vi "Main.vi"(10 "Ip-Address":string="192.168.81.153", 11 "Module Admin":refnum<class "Delacor_lib_QMH_Cloneable Module Admin.lvclass">) -> ()   [LabVIEW 2021, in "RT Acquisition Engine.lvlib"]
doc: "This template is based off of the Queued Message Handler design pattern and the Queued Message Handler project template that ships with LabVIEW.\n\nThe main difference is that the queue is private to this module and communication between modules is performed via Broadcast and Request events.\n\nRequest events are wrapped in public API methods and are handled in the Event Handling Loop (EHL) of this VI. Any module can register for Broadcast events sent by this module. The EHL generates messages based on user interface actions.\n\nThe Message Handling Loop (MHL) processes messages generated by the EHL, or by other messages. The messages are string values, so new messages can be added easily to the Message Cases case structure in the MHL. Each message cluster can also provide an optional value for Message Data, which is a variant that can be converted to whatever message-specific data is required.\n_____\nBased on DQMH Project Template 7.0.1.1316."
uses:
  RT Acquisition Engine.lvlib
  <vilib>/Delacor/Delacor QMH/Libraries/Cloneable Module Admin_class/Delacor_lib_QMH_Cloneable Module Admin.lvclass
  C:/Program Files (x86)/National Instruments/LabVIEW 2024/vi.lib/Delacor/Delacor QMH/Libraries/Module Admin_class/Delacor_lib_QMH_Module Admin.lvclass
  Analog Output/Controls/AO JSON Data Cluster.ctl
  Analog Output/Controls/AO Interface Data Cluster.ctl
  Analog Output/Controls/AO Channel Configuration Cluster.ctl
  Analog Output/Controls/AO Timing Cluster.ctl
  Digital Output/Controls/DIO Configuration cluster.ctl
  Digital Output/Controls/DIO Interface Data.ctl
  Digital Output/SubVIs/Digital Dynamic Cluster.ctl
  Host/Async JSON Cluster.ctl
  Host/Async Interface Data Cluster.ctl
  Async Serial/Controls/Async Serial Configuration Cluster.ctl
  Async Serial/Controls/Async Frame Info Cluster.ctl
  Async Serial/Controls/Async Message Info Cluster.ctl
  Host-Control's/TCP Tx-Rx cluster.ctl
  Host-Control's/AI-Data from RT.ctl
  Main Engine/Controls/Main Engine Serial Info JSON Data.ctl
  Main Engine/Controls/Main Engine DAQ Harware Info JSON Data.ctl
  Main Engine/Controls/Main Engine Ehernet IP Address JSON Data.ctl
  Module Data--cluster.ctl
  Hardware Info (Reply Payload)--cluster.ctl
  Host-Control's/RT Data's.ctl
  Host-Control's/DIO Data's from RT.ctl
  <vilib>/Wovalab/Utilities/Helper Loop Periodic Timing/Helper Loop Periodic Timing.lvclass/Helper Loop Periodic Timing.ctl
  <vilib>/Delacor/Delacor QMH/Libraries/Message Queue_class/Delacor_lib_QMH_Message Queue.lvclass/Delacor_lib_QMH_Message Queue.ctl
  <vilib>/Delacor/Delacor QMH/Libraries/Cloneable Module Admin_class/Delacor_lib_QMH_Cloneable Module Admin.lvclass/Delacor_lib_QMH_Cloneable Module Admin.ctl
  Stop Argument--cluster.ctl
  <vilib>/Delacor/Delacor QMH/Libraries/Module Admin_class/Delacor_lib_QMH_Module Admin.lvclass/Delacor_lib_QMH_Module Admin.ctl
  Write Data To the RT Argument--cluster.ctl
  <vilib>/Utility/miscctls.llb/LVPointTypeDef.ctl
  <vilib>/Delacor/Delacor QMH/Libraries/Message Queue_class/Delacor_lib_QMH_Enqueue Message (Single).vi
  <vilib>/Delacor/Delacor QMH/Libraries/Cloneable Module Admin_class/Delacor_lib_QMH_Get Module ID.vi
  <vilib>/Delacor/Delacor QMH/Libraries/Module Admin_class/Delacor_lib_QMH_Get External Launch.vi
  <vilib>/Wovalab/Utilities/Helper Loop Periodic Timing/U32 Max Value--constant.vi
  <vilib>/Wovalab/Utilities/Helper Loop Periodic Timing/Update Last Execution Time.vi
  <vilib>/Wovalab/Utilities/Helper Loop Periodic Timing/Helper Loop Periodic Timing.lvclass
  <vilib>/Delacor/Delacor QMH/Libraries/Message Queue_class/Delacor_lib_QMH_Message Queue.lvclass
  TCP-IP Engine/TCP-IP Engine.lvlib
  <vilib>/addons/_JKI.lib/Serialization/JSON/JKI JSON Serialization.lvlib
panel:
  in  "AI-Info":T1
  out "TCP-IP Data Out 2":string
  out "Connection Status?":bool
  out "TCP-IP Module ID":i32
  out "data":T2={"Interface"="CPU", "Command"="CPU Info", "SubCmd"="Monitor", "Data"=variant}
  in  "DO":T3={"Interface"="DIO", "Interface Data"={"Command"="Configure", "SubCmd"="DO", "Frequency"=500, "Data"=[{"Channel"="Mod1/port0/line0", "Data"=[0], "Identification Name"=""}, {"Channel"="Mod1/port0/line1", "Data"=[0], "Identification Name"=""}, {"Channel"="Mod1/port0/line2", "Data"=[0], "Identification Name"=""}, {"Channel"="Mod1/port0/line3", "Data"=[0], "Identification Name"=""}, {"Channel"="Mod1/port0/line4", "Data"=[0], "Identification Name"=""}, {"Channel"="Mod1/port0/line5", "Data"=[0], "Identification Name"=""}, {"Channel"="Mod1/port0/line6", "Data"=[0], "Identification Name"=""}, {"Channel"="Mod1/port0/line7", "Data"=[0], "Identification Name"=""}, {"Channel"="Mod1/port0/line8", "Data"=[0], "Identification Name"=""}, {"Channel"="Mod1/port0/line9", "Data"=[0], "Identification Name"=""}, {"Channel"="Mod1/port0/line10", "Data"=[0], "Identification Name"=""}, {"Channel"="Mod1/port0/line11", "Data"=[0], "Identification Name"=""}, {"Channel"="Mod1/port0/line12", "Data"=[0], "Identification Name"=""}, {"Channel"="Mod1/port0/line13", "Data"=[0], "Identification Name"=""}, {"Channel"="Mod1/port0/line14", "Data"=[0], "Identification Name"=""}, {"Channel"="Mod1/port0/line15", "Data"=[0], "Identification Name"=""}, {"Channel"="Mod1/port0/line16", "Data"=[0], "Identification Name"=""}, {"Channel"="Mod1/port0/line17", "Data"=[0], "Identification Name"=""}, {"Channel"="Mod1/port0/line18", "Data"=[0], "Identification Name"=""}, {"Channel"="Mod1/port0/line19", "Data"=[0], "Identification Name"=""}, {"Channel"="Mod1/port0/line20", "Data"=[0], "Identification Name"=""}, {"Channel"="Mod1/port0/line21", "Data"=[0], "Identification Name"=""}, {"Channel"="Mod1/port0/line22", "Data"=[0], "Identification Name"=""}, {"Channel"="Mod1/port0/line23", "Data"=[0], "Identification Name"=""}, {"Channel"="Mod1/port0/line24", "Data"=[0], "Identification Name"=""}, {"Channel"="Mod1/port0/line25", "Data"=[0], "Identification Name"=""}, {"Channel"="Mod1/port0/line26", "Data"=[0], "Identification Name"=""}, {"Channel"="Mod1/port0/line27", "Data"=[0], "Identification Name"=""}, {"Channel"="Mod1/port0/line28", "Data"=[0], "Identification Name"=""}, {"Channel"="Mod1/port0/line29", "Data"=[0], "Identification Name"=""}, {"Channel"="Mod1/port0/line30", "Data"=[0], "Identification Name"=""}, {"Channel"="Mod1/port0/line31", "Data"=[0], "Identification Name"=""}]}}
  in  "Channel Data":cluster{"AI":T6, "DI":T3, "DO":T3, "Async":T10}={"AI"={"Interface"="AIO", "Interface Data"={"Command"="Configure", "SubCmd"="AI", "Data"=[{"Channel"="Mod2/ai0", "Min Value"=-5.0, "Max Value"=5.0, "Type"="Voltage", "Terminal Configure"=10083, "Dynamic"=0, "Dyn Type"="", "Data"=[], "File Name"="", "Column"=0, "Frequency"=0.0}, {"Channel"="Mod2/ai1", "Min Value"=-5.0, "Max Value"=5.0, "Type"="Voltage", "Terminal Configure"=10083, "Dynamic"=0, "Dyn Type"="", "Data"=[], "File Name"="", "Column"=0, "Frequency"=0.0}, {"Channel"="Mod2/ai2", "Min Value"=-5.0, "Max Value"=5.0, "Type"="Voltage", "Terminal Configure"=10083, "Dynamic"=0, "Dyn Type"="", "Data"=[], "File Name"="", "Column"=0, "Frequency"=0.0}, {"Channel"="Mod2/ai3", "Min Value"=-5.0, "Max Value"=5.0, "Type"="Voltage", "Terminal Configure"=10083, "Dynamic"=0, "Dyn Type"="", "Data"=[], "File Name"="", "Column"=0, "Frequency"=0.0}, {"Channel"="Mod2/ai4", "Min Value"=-5.0, "Max Value"=5.0, "Type"="Voltage", "Terminal Configure"=10083, "Dynamic"=0, "Dyn Type"="", "Data"=[], "File Name"="", "Column"=0, "Frequency"=0.0}, {"Channel"="Mod2/ai5", "Min Value"=-5.0, "Max Value"=5.0, "Type"="Voltage", "Terminal Configure"=10083, "Dynamic"=0, "Dyn Type"="", "Data"=[], "File Name"="", "Column"=0, "Frequency"=0.0}, {"Channel"="Mod2/ai6", "Min Value"=-5.0, "Max Value"=5.0, "Type"="Voltage", "Terminal Configure"=10083, "Dynamic"=0, "Dyn Type"="", "Data"=[], "File Name"="", "Column"=0, "Frequency"=0.0}, {"Channel"="Mod2/ai7", "Min Value"=-5.0, "Max Value"=5.0, "Type"="Voltage", "Terminal Configure"=10083, "Dynamic"=0, "Dyn Type"="", "Data"=[], "File Name"="", "Column"=0, "Frequency"=0.0}, {"Channel"="Mod2/ai8", "Min Value"=-5.0, "Max Value"=5.0, "Type"="Voltage", "Terminal Configure"=10083, "Dynamic"=0, "Dyn Type"="", "Data"=[], "File Name"="", "Column"=0, "Frequency"=0.0}, {"Channel"="Mod2/ai9", "Min Value"=-5.0, "Max Value"=5.0, "Type"="Voltage", "Terminal Configure"=10083, "Dynamic"=0, "Dyn Type"="", "Data"=[], "File Name"="", "Column"=0, "Frequency"=0.0}, {"Channel"="Mod2/ai10", "Min Value"=-5.0, "Max Value"=5.0, "Type"="Voltage", "Terminal Configure"=10083, "Dynamic"=0, "Dyn Type"="", "Data"=[], "File Name"="", "Column"=0, "Frequency"=0.0}, {"Channel"="Mod2/ai11", "Min Value"=-5.0, "Max Value"=5.0, "Type"="Voltage", "Terminal Configure"=10083, "Dynamic"=0, "Dyn Type"="", "Data"=[], "File Name"="", "Column"=0, "Frequency"=0.0}, {"Channel"="Mod2/ai12", "Min Value"=-5.0, "Max Value"=5.0, "Type"="Voltage", "Terminal Configure"=10083, "Dynamic"=0, "Dyn Type"="", "Data"=[], "File Name"="", "Column"=0, "Frequency"=0.0}, {"Channel"="Mod2/ai13", "Min Value"=-5.0, "Max Value"=5.0, "Type"="Voltage", "Terminal Configure"=10083, "Dynamic"=0, "Dyn Type"="", "Data"=[], "File Name"="", "Column"=0, "Frequency"=0.0}, {"Channel"="Mod2/ai14", "Min Value"=-5.0, "Max Value"=5.0, "Type"="Voltage", "Terminal Configure"=10083, "Dynamic"=0, "Dyn Type"="", "Data"=[], "File Name"="", "Column"=0, "Frequency"=0.0}, {"Channel"="Mod2/ai15", "Min Value"=-5.0, "Max Value"=5.0, "Type"="Voltage", "Terminal Configure"=10083, "Dynamic"=0, "Dyn Type"="", "Data"=[], "File Name"="", "Column"=0, "Frequency"=0.0}, {"Channel"="Mod2/ai16", "Min Value"=-5.0, "Max Value"=5.0, "Type"="Voltage", "Terminal Configure"=10083, "Dynamic"=0, "Dyn Type"="", "Data"=[], "File Name"="", "Column"=0, "Frequency"=0.0}, {"Channel"="Mod2/ai17", "Min Value"=-5.0, "Max Value"=5.0, "Type"="Voltage", "Terminal Configure"=10083, "Dynamic"=0, "Dyn Type"="", "Data"=[], "File Name"="", "Column"=0, "Frequency"=0.0}, {"Channel"="Mod2/ai18", "Min Value"=-5.0, "Max Value"=5.0, "Type"="Voltage", "Terminal Configure"=10083, "Dynamic"=0, "Dyn Type"="", "Data"=[], "File Name"="", "Column"=0, "Frequency"=0.0}, {"Channel"="Mod2/ai19", "Min Value"=-5.0, "Max Value"=5.0, "Type"="Voltage", "Terminal Configure"=10083, "Dynamic"=0, "Dyn Type"="", "Data"=[], "File Name"="", "Column"=0, "Frequency"=0.0}, {"Channel"="Mod2/ai20", "Min Value"=-5.0, "Max Value"=5.0, "Type"="Voltage", "Terminal Configure"=10083, "Dynamic"=0, "Dyn Type"="", "Data"=[], "File Name"="", "Column"=0, "Frequency"=0.0}, {"Channel"="Mod2/ai21", "Min Value"=-5.0, "Max Value"=5.0, "Type"="Voltage", "Terminal Configure"=10083, "Dynamic"=0, "Dyn Type"="", "Data"=[], "File Name"="", "Column"=0, "Frequency"=0.0}, {"Channel"="Mod2/ai22", "Min Value"=-5.0, "Max Value"=5.0, "Type"="Voltage", "Terminal Configure"=10083, "Dynamic"=0, "Dyn Type"="", "Data"=[], "File Name"="", "Column"=0, "Frequency"=0.0}, {"Channel"="Mod2/ai23", "Min Value"=-5.0, "Max Value"=5.0, "Type"="Voltage", "Terminal Configure"=10083, "Dynamic"=0, "Dyn Type"="", "Data"=[], "File Name"="", "Column"=0, "Frequency"=0.0}, {"Channel"="Mod2/ai24", "Min Value"=-5.0, "Max Value"=5.0, "Type"="Voltage", "Terminal Configure"=10083, "Dynamic"=0, "Dyn Type"="", "Data"=[], "File Name"="", "Column"=0, "Frequency"=0.0}, {"Channel"="Mod2/ai25", "Min Value"=-5.0, "Max Value"=5.0, "Type"="Voltage", "Terminal Configure"=10083, "Dynamic"=0, "Dyn Type"="", "Data"=[], "File Name"="", "Column"=0, "Frequency"=0.0}, {"Channel"="Mod2/ai26", "Min Value"=-5.0, "Max Value"=5.0, "Type"="Voltage", "Terminal Configure"=10083, "Dynamic"=0, "Dyn Type"="", "Data"=[], "File Name"="", "Column"=0, "Frequency"=0.0}, {"Channel"="Mod2/ai27", "Min Value"=-5.0, "Max Value"=5.0, "Type"="Voltage", "Terminal Configure"=10083, "Dynamic"=0, "Dyn Type"="", "Data"=[], "File Name"="", "Column"=0, "Frequency"=0.0}, {"Channel"="Mod2/ai28", "Min Value"=-5.0, "Max Value"=5.0, "Type"="Voltage", "Terminal Configure"=10083, "Dynamic"=0, "Dyn Type"="", "Data"=[], "File Name"="", "Column"=0, "Frequency"=0.0}, {"Channel"="Mod2/ai29", "Min Value"=-5.0, "Max Value"=5.0, "Type"="Voltage", "Terminal Configure"=10083, "Dynamic"=0, "Dyn Type"="", "Data"=[], "File Name"="", "Column"=0, "Frequency"=0.0}, {"Channel"="Mod2/ai30", "Min Value"=-5.0, "Max Value"=5.0, "Type"="Voltage", "Terminal Configure"=10083, "Dynamic"=0, "Dyn Type"="", "Data"=[], "File Name"="", "Column"=0, "Frequency"=0.0}, {"Channel"="Mod2/ai31", "Min Value"=-5.0, "Max Value"=5.0, "Type"="Voltage", "Terminal Configure"=65535, "Dynamic"=0, "Dyn Type"="", "Data"=[], "File Name"="", "Column"=0, "Frequency"=0.0}], "Timing"={"samples per channel"=4, "sample mode"=10123, "Sampling Rate"=2.0}}}, "DI"={"Interface"="DIO", "Interface Data"={"Command"="Configure", "SubCmd"="DI", "Frequency"=500, "Data"=[{"Channel"="Mod3/port0/line0", "Data"=[0], "Identification Name"=""}, {"Channel"="Mod3/port0/line1", "Data"=[0], "Identification Name"=""}, {"Channel"="Mod3/port0/line2", "Data"=[0], "Identification Name"=""}, {"Channel"="Mod3/port0/line3", "Data"=[0], "Identification Name"=""}, {"Channel"="Mod3/port0/line4", "Data"=[0], "Identification Name"=""}, {"Channel"="Mod3/port0/line5", "Data"=[0], "Identification Name"=""}, {"Channel"="Mod3/port0/line6", "Data"=[0], "Identification Name"=""}, {"Channel"="Mod3/port0/line7", "Data"=[0], "Identification Name"=""}, {"Channel"="Mod3/port0/line8", "Data"=[0], "Identification Name"=""}, {"Channel"="Mod3/port0/line9", "Data"=[0], "Identification Name"=""}, {"Channel"="Mod3/port0/line10", "Data"=[0], "Identification Name"=""}, {"Channel"="Mod3/port0/line11", "Data"=[0], "Identification Name"=""}, {"Channel"="Mod3/port0/line12", "Data"=[0], "Identification Name"=""}, {"Channel"="Mod3/port0/line13", "Data"=[0], "Identification Name"=""}, {"Channel"="Mod3/port0/line14", "Data"=[0], "Identification Name"=""}, {"Channel"="Mod3/port0/line15", "Data"=[0], "Identification Name"=""}, {"Channel"="Mod3/port0/line16", "Data"=[0], "Identification Name"=""}, {"Channel"="Mod3/port0/line17", "Data"=[0], "Identification Name"=""}, {"Channel"="Mod3/port0/line18", "Data"=[0], "Identification Name"=""}, {"Channel"="Mod3/port0/line19", "Data"=[0], "Identification Name"=""}, {"Channel"="Mod3/port0/line20", "Data"=[0], "Identification Name"=""}, {"Channel"="Mod3/port0/line21", "Data"=[0], "Identification Name"=""}, {"Channel"="Mod3/port0/line22", "Data"=[0], "Identification Name"=""}, {"Channel"="Mod3/port0/line23", "Data"=[0], "Identification Name"=""}, {"Channel"="Mod3/port0/line24", "Data"=[0], "Identification Name"=""}, {"Channel"="Mod3/port0/line25", "Data"=[0], "Identification Name"=""}, {"Channel"="Mod3/port0/line26", "Data"=[0], "Identification Name"=""}, {"Channel"="Mod3/port0/line27", "Data"=[0], "Identification Name"=""}, {"Channel"="Mod3/port0/line28", "Data"=[0], "Identification Name"=""}, {"Channel"="Mod3/port0/line29", "Data"=[0], "Identification Name"=""}, {"Channel"="Mod3/port0/line30", "Data"=[0], "Identification Name"=""}, {"Channel"="Mod3/port0/line31", "Data"=[0], "Identification Name"=""}, {"Channel"="Mod4/port0/line0", "Data"=[0], "Identification Name"=""}, {"Channel"="Mod4/port0/line1", "Data"=[0], "Identification Name"=""}, {"Channel"="Mod4/port0/line2", "Data"=[0], "Identification Name"=""}, {"Channel"="Mod4/port0/line3", "Data"=[0], "Identification Name"=""}, {"Channel"="Mod4/port0/line4", "Data"=[0], "Identification Name"=""}, {"Channel"="Mod4/port0/line5", "Data"=[0], "Identification Name"=""}, {"Channel"="Mod4/port0/line6", "Data"=[0], "Identification Name"=""}, {"Channel"="Mod4/port0/line7", "Data"=[0], "Identification Name"=""}, {"Channel"="Mod4/port0/line8", "Data"=[0], "Identification Name"=""}, {"Channel"="Mod4/port0/line9", "Data"=[0], "Identification Name"=""}, {"Channel"="Mod4/port0/line10", "Data"=[0], "Identification Name"=""}, {"Channel"="Mod4/port0/line11", "Data"=[0], "Identification Name"=""}, {"Channel"="Mod4/port0/line12", "Data"=[0], "Identification Name"=""}, {"Channel"="Mod4/port0/line13", "Data"=[0], "Identification Name"=""}, {"Channel"="Mod4/port0/line14", "Data"=[0], "Identification Name"=""}, {"Channel"="Mod4/port0/line15", "Data"=[0], "Identification Name"=""}, {"Channel"="Mod4/port0/line16", "Data"=[0], "Identification Name"=""}, {"Channel"="Mod4/port0/line17", "Data"=[0], "Identification Name"=""}, {"Channel"="Mod4/port0/line18", "Data"=[0], "Identification Name"=""}, {"Channel"="Mod4/port0/line19", "Data"=[0], "Identification Name"=""}, {"Channel"="Mod4/port0/line20", "Data"=[0], "Identification Name"=""}, {"Channel"="Mod4/port0/line21", "Data"=[0], "Identification Name"=""}, {"Channel"="Mod4/port0/line22", "Data"=[0], "Identification Name"=""}, {"Channel"="Mod4/port0/line23", "Data"=[0], "Identification Name"=""}, {"Channel"="Mod4/port0/line24", "Data"=[0], "Identification Name"=""}, {"Channel"="Mod4/port0/line25", "Data"=[0], "Identification Name"=""}, {"Channel"="Mod4/port0/line26", "Data"=[0], "Identification Name"=""}, {"Channel"="Mod4/port0/line27", "Data"=[0], "Identification Name"=""}, {"Channel"="Mod4/port0/line28", "Data"=[0], "Identification Name"=""}, {"Channel"="Mod4/port0/line29", "Data"=[0], "Identification Name"=""}, {"Channel"="Mod4/port0/line30", "Data"=[0], "Identification Name"=""}, {"Channel"="Mod4/port0/line31", "Data"=[0], "Identification Name"=""}]}}, "DO"={"Interface"="DIO", "Interface Data"={"Command"="Configure", "SubCmd"="DO", "Frequency"=500, "Data"=[{"Channel"="Mod1/port0/line0", "Data"=[0], "Identification Name"=""}, {"Channel"="Mod1/port0/line1", "Data"=[0], "Identification Name"=""}, {"Channel"="Mod1/port0/line2", "Data"=[0], "Identification Name"=""}, {"Channel"="Mod1/port0/line3", "Data"=[0], "Identification Name"=""}, {"Channel"="Mod1/port0/line4", "Data"=[0], "Identification Name"=""}, {"Channel"="Mod1/port0/line5", "Data"=[0], "Identification Name"=""}, {"Channel"="Mod1/port0/line6", "Data"=[0], "Identification Name"=""}, {"Channel"="Mod1/port0/line7", "Data"=[0], "Identification Name"=""}, {"Channel"="Mod1/port0/line8", "Data"=[0], "Identification Name"=""}, {"Channel"="Mod1/port0/line9", "Data"=[0], "Identification Name"=""}, {"Channel"="Mod1/port0/line10", "Data"=[0], "Identification Name"=""}, {"Channel"="Mod1/port0/line11", "Data"=[0], "Identification Name"=""}, {"Channel"="Mod1/port0/line12", "Data"=[0], "Identification Name"=""}, {"Channel"="Mod1/port0/line13", "Data"=[0], "Identification Name"=""}, {"Channel"="Mod1/port0/line14", "Data"=[0], "Identification Name"=""}, {"Channel"="Mod1/port0/line15", "Data"=[0], "Identification Name"=""}, {"Channel"="Mod1/port0/line16", "Data"=[0], "Identification Name"=""}, {"Channel"="Mod1/port0/line17", "Data"=[0], "Identification Name"=""}, {"Channel"="Mod1/port0/line18", "Data"=[0], "Identification Name"=""}, {"Channel"="Mod1/port0/line19", "Data"=[0], "Identification Name"=""}, {"Channel"="Mod1/port0/line20", "Data"=[0], "Identification Name"=""}, {"Channel"="Mod1/port0/line21", "Data"=[0], "Identification Name"=""}, {"Channel"="Mod1/port0/line22", "Data"=[0], "Identification Name"=""}, {"Channel"="Mod1/port0/line23", "Data"=[0], "Identification Name"=""}, {"Channel"="Mod1/port0/line24", "Data"=[0], "Identification Name"=""}, {"Channel"="Mod1/port0/line25", "Data"=[0], "Identification Name"=""}, {"Channel"="Mod1/port0/line26", "Data"=[0], "Identification Name"=""}, {"Channel"="Mod1/port0/line27", "Data"=[0], "Identification Name"=""}, {"Channel"="Mod1/port0/line28", "Data"=[0], "Identification Name"=""}, {"Channel"="Mod1/port0/line29", "Data"=[0], "Identification Name"=""}, {"Channel"="Mod1/port0/line30", "Data"=[0], "Identification Name"=""}, {"Channel"="Mod1/port0/line31", "Data"=[0], "Identification Name"=""}]}}, "Async"={"Interface"="Async", "Interface Data"={"Command"="Configure", "SubCmd"="Async", "Data"=[{"Port"="com10", "Minor Frame Freq"=200, "Minor Frame Count"=1, "Frame Info"=[{"Frame ID"=1, "Message Info"=[{"Message"=[1], "Message Name"="m1"}]}], "Sensor Type"=0, "OIM Address"=0}]}}} {"Async"."Interface Data"."Data"."Minor Frame Count" min=5 max=8 step=1; "AI"."Interface Data"."Timing"."sample mode" items=["Finite Samples"=10178, "Continuous Samples"=10123, "Hardware Timed Single Point"=12522]}
  out "error out":errorcluster
  out "Status":string
  in  "Simulate EHL Error":bool
  in  "Simulate MHL Error":bool
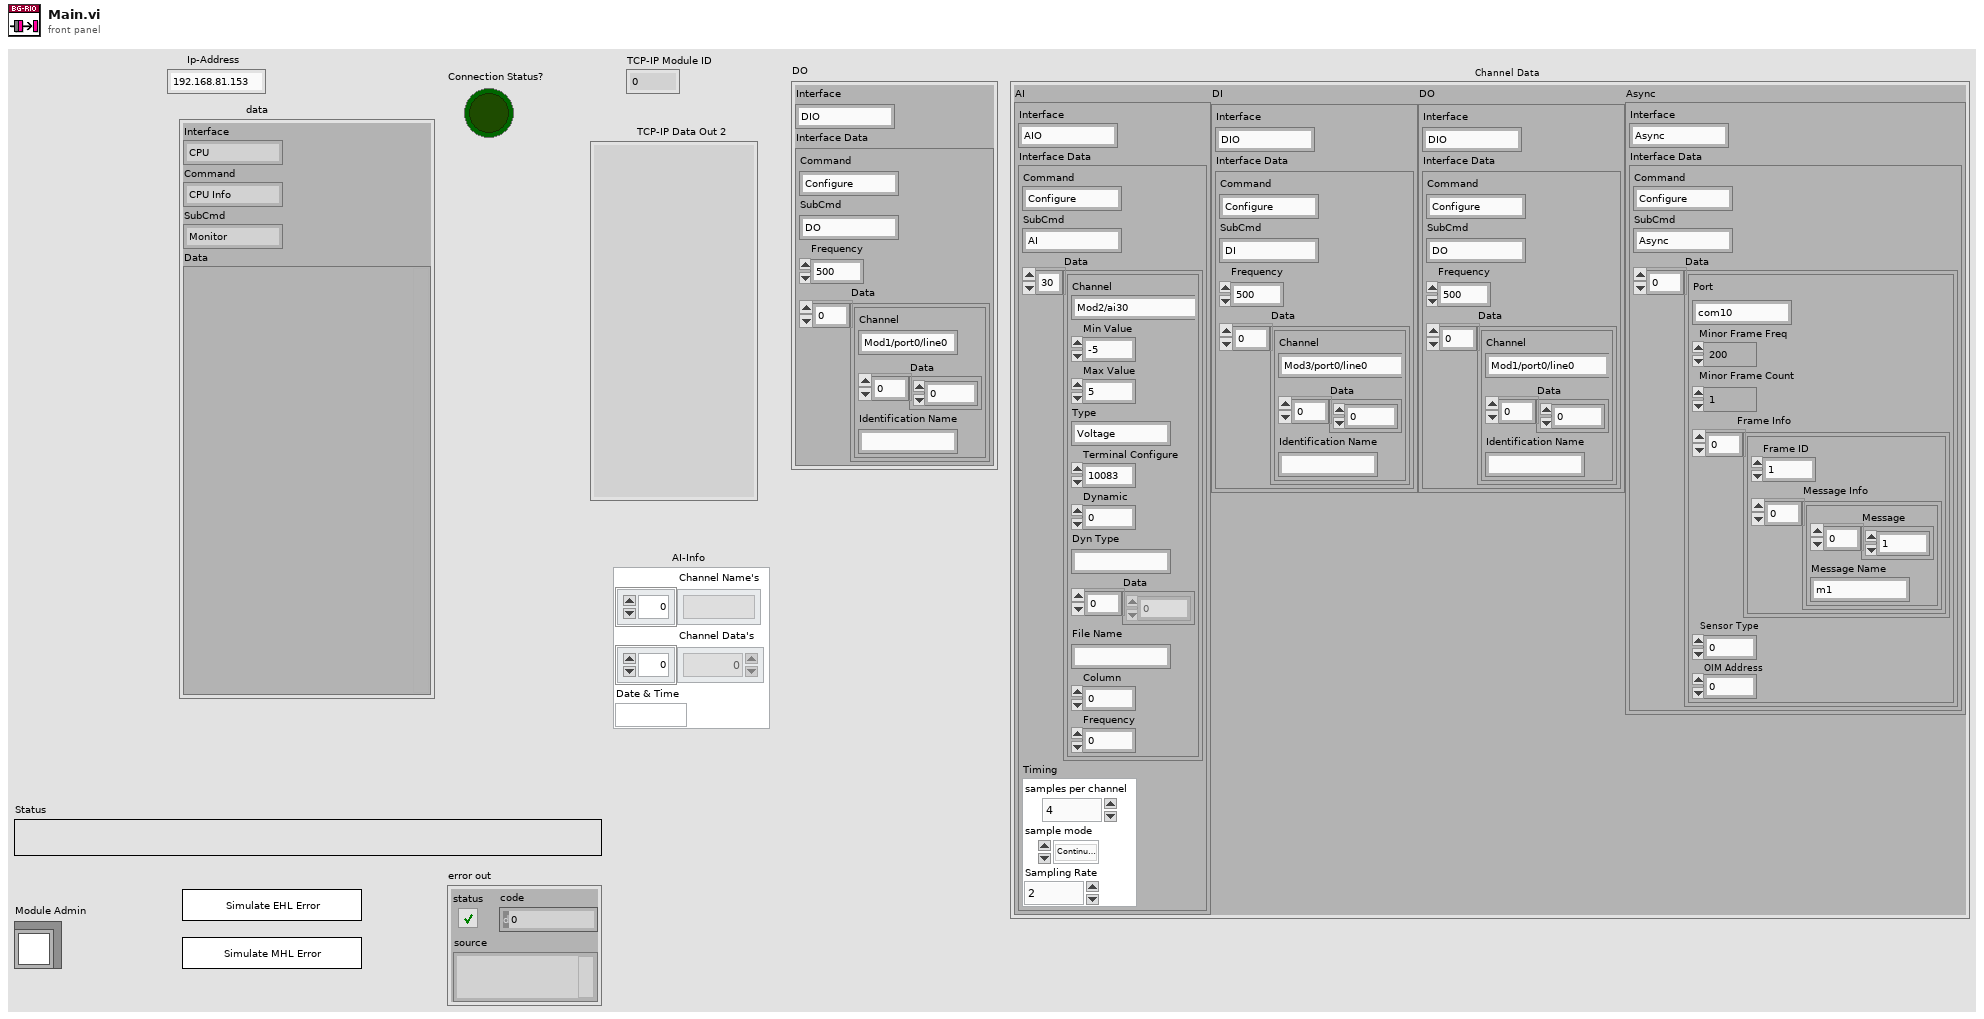
[diagram p1: front panel]
types:
  T1 = typedef "AI-Data from RT.ctl" = cluster{"Channel Name's":string[], "Channel Data's":dbl[], "Date & Time":string}
  T2 = typedef "TCP Tx-Rx cluster.ctl" = cluster{"Interface":string, "Command":string, "SubCmd":string, "Data":variant}
  T3 = typedef "DIO Configuration cluster.ctl" = cluster{"Interface":string, "Interface Data":T4}
  T4 = typedef "DIO Interface Data.ctl" = cluster{"Command":string, "SubCmd":string, "Frequency":u16, "Data":T5[]}
  T5 = typedef "Digital Dynamic Cluster.ctl" = cluster{"Channel":string, "Data":u8[], "Identification Name":string}
  T6 = typedef "AO JSON Data Cluster.ctl" = cluster{"Interface":string, "Interface Data":T7}
  T7 = typedef "AO Interface Data Cluster.ctl" = cluster{"Command":string, "SubCmd":string, "Data":T8[], "Timing":T9}
  T8 = typedef "AO Channel Configuration Cluster.ctl" = cluster{"Channel":string, "Min Value":dbl, "Max Value":dbl, "Type":string, "Terminal Configure":u16, "Dynamic":u8, "Dyn Type":string, "Data":dbl[], "File Name":string, "Column":i32, "Frequency":dbl}
  T9 = typedef "AO Timing Cluster.ctl" = cluster{"samples per channel":i32, "sample mode":i32, "Sampling Rate":dbl}
  T10 = typedef "Async JSON Cluster.ctl" = cluster{"Interface":string, "Interface Data":T11}
  T11 = typedef "Async Interface Data Cluster.ctl" = cluster{"Command":string, "SubCmd":string, "Data":T12[]}
  T12 = typedef "Async Serial Configuration Cluster.ctl" = cluster{"Port":string, "Minor Frame Freq":u16, "Minor Frame Count":u16, "Frame Info":T13[], "Sensor Type":u16, "OIM Address":u16}
  T13 = typedef "Async Frame Info Cluster.ctl" = cluster{"Frame ID":u16, "Message Info":T14[]}
  T14 = typedef "Async Message Info Cluster.ctl" = cluster{"Message":u8[], "Message Name":string}
  T15 = typedef "Main Engine Serial Info JSON Data.ctl" = cluster{"Command":string, "SubCmd":string, "Channel":string[]}
  T16 = typedef "Main Engine DAQ Harware Info JSON Data.ctl" = cluster{"Command":string, "SubCmd":string, "Input":string[], "Output":string[]}
  T17 = typedef "Main Engine Ehernet IP Address JSON Data.ctl" = cluster{"Command":string, "SubCmd":string, "IP":string[]}
  T18 = cluster{"Serial Hardware Info JSON Format":T15, "Hardware Info JSON Format":T16, "Hardware Info JSON Format":T16, "Ethernet IP Address JSON Format":T17}
  T19 = typedef "RT Acquisition Engine.lvlib/Request Events--cluster.ctl" = cluster{"Stop Module":refnum<user-event>, "Show Panel":refnum<user-event>, "Hide Panel":refnum<user-event>, "Show Diagram":refnum<user-event>, "Get Module Execution Status":refnum<user-event>, "Write Data To the RT":refnum<user-event>, "Hardware Info":refnum<user-event>}
  T20 = enum16{"Standard", "Buffered", "CRLF", "Immediate"}
  T21 = enum32{"invalid lock state", "Not Locked", "Locked (No Password)", "Password-protected"}
  T22 = typedef "RT Acquisition Engine.lvlib/Stop Argument--cluster.ctl" = cluster{"Module ID":i32, "Origin":string, "Exit via Stop Module Req?":bool, "Wait for Module to stop?":bool}
  T23 = typedef "RT Acquisition Engine.lvlib/Write Data To the RT Argument--cluster.ctl" = cluster{"Module ID":i32, "Data In":string}
  T24 = typedef "LVPointTypeDef.ctl" = cluster{"Horizontal":i16, "Vertical":i16}
  T25 = enum32{"Invalid", "Standard", "Closed", "Hidden", "Minimized", "Maximized"}
  T26 = typedef "RT Acquisition Engine.lvlib/Hardware Info (Reply Payload)--cluster.ctl" = cluster{"Module ID":i32, "Hardware Information":variant, "error":errorcluster}
  T27 = typedef "RT Acquisition Engine.lvlib/Module Data--cluster.ctl" = cluster{"Status":string, "This Module ID":i32, "RT-IP":string, "Hardware Info Request Ref":cluster{"Wait Notifier":refnum<notifier>, "wait for reply":bool}, "RT-Data's":T28, "Connection Status?":bool}
  T28 = typedef "RT Data's.ctl" = cluster{"DO Info":T29, "AI-Data From RT--Cluster":T1, "Hardware Information":variant}
  T29 = typedef "DIO Data's from RT.ctl" = cluster{"Channels":string[], "Data":bool[], "Time":string}
  T30 = typedef "TCP-IP Engine.lvlib/Broadcast Events--cluster.ctl" = cluster{"Module Did Init":refnum<user-event>, "Status Updated":refnum<user-event>, "Error Reported":refnum<user-event>, "Module Did Stop":refnum<user-event>, "Update Module Execution Status":refnum<user-event>, "Open Connection Status":refnum<user-event>, "TCP-Read Data Out":refnum<user-event>}
  T31 = cluster{"Wait Notifier":refnum<notifier>, "wait for reply":bool}
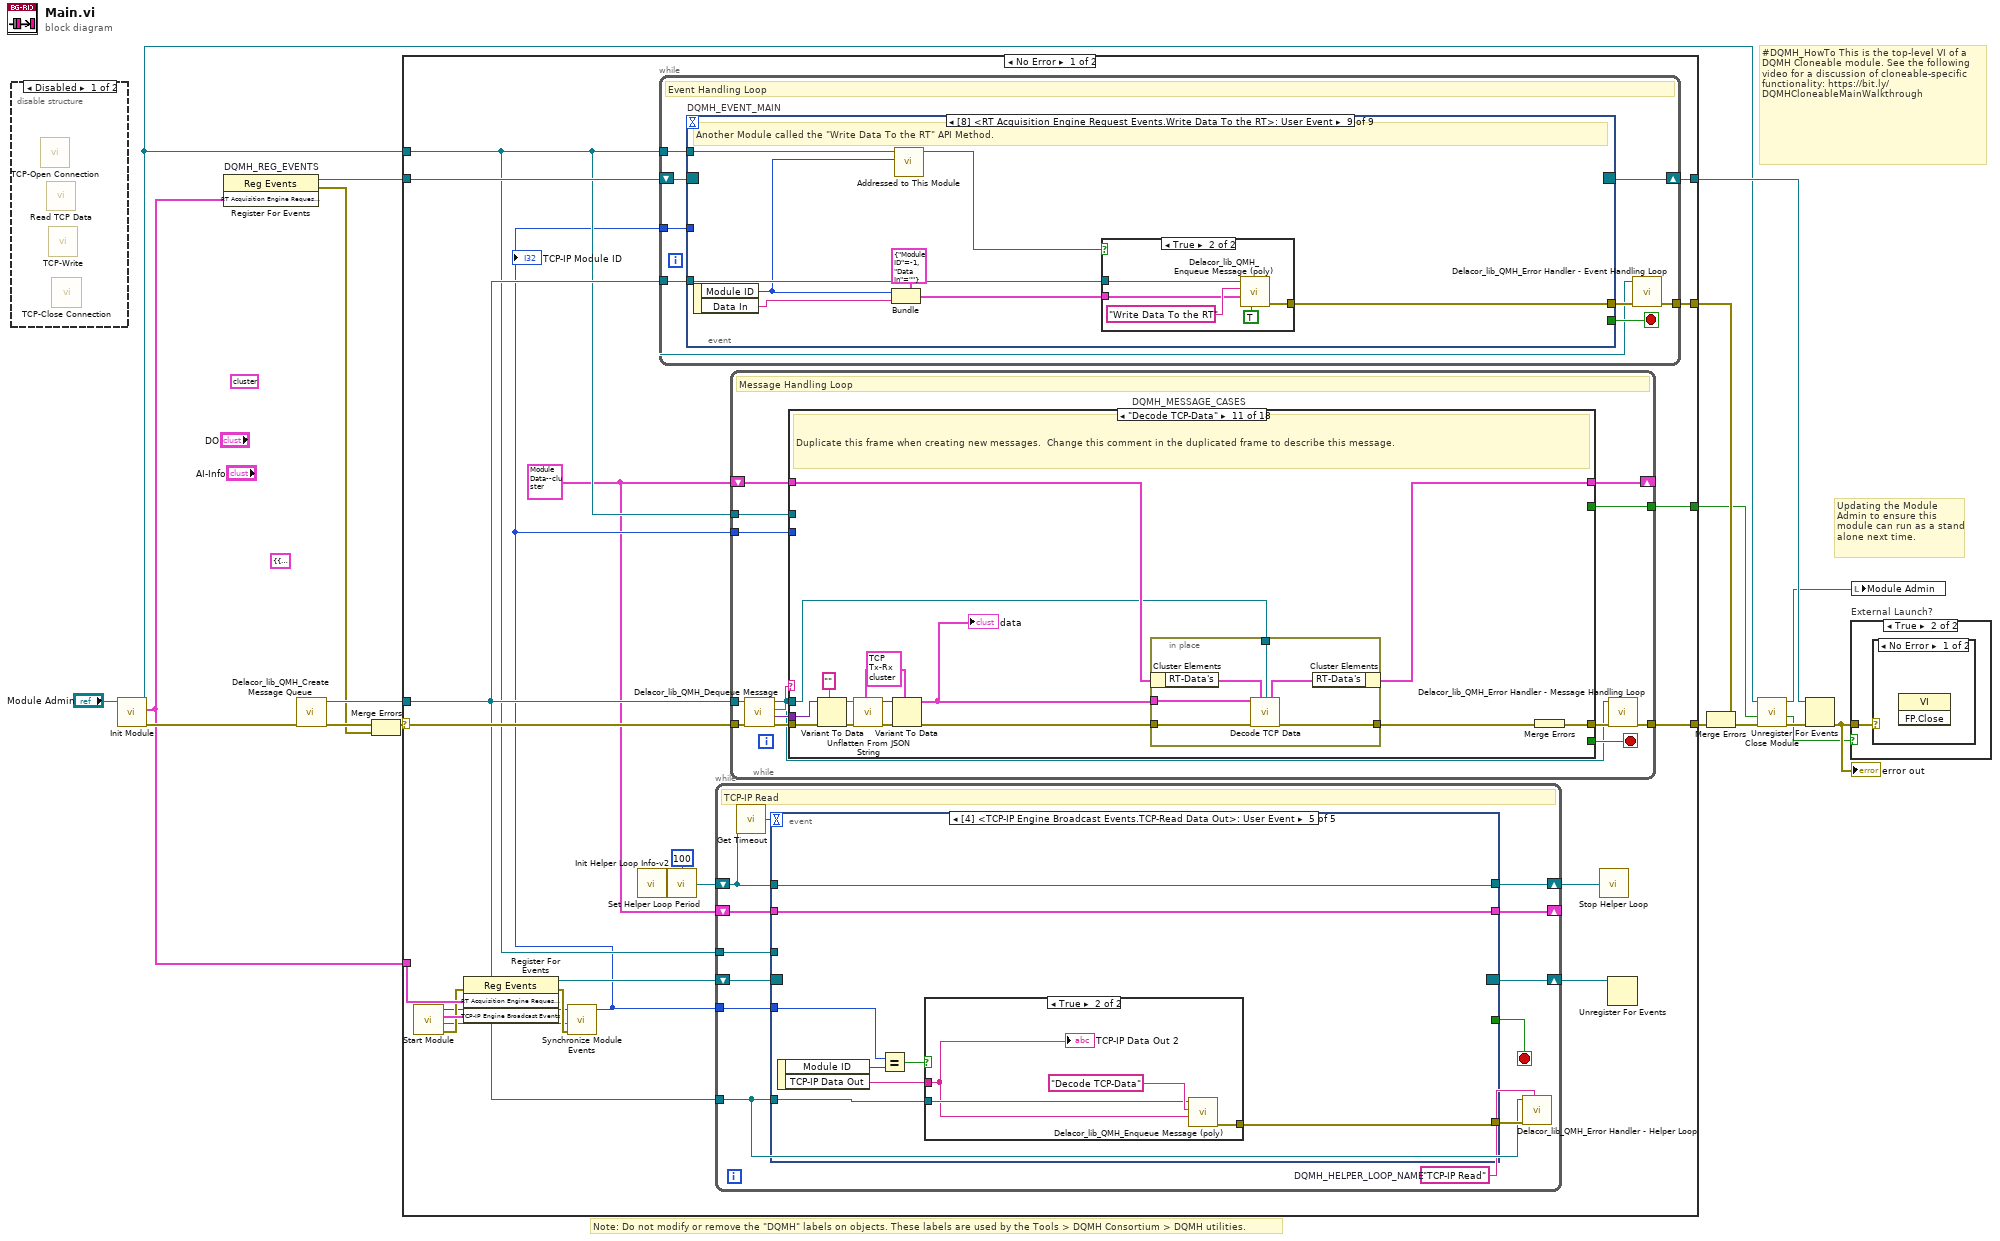
[diagram p0: block diagram]
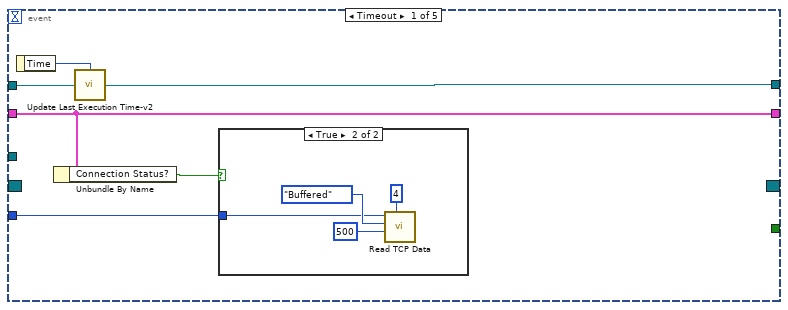
[diagram p3: hidden frame]
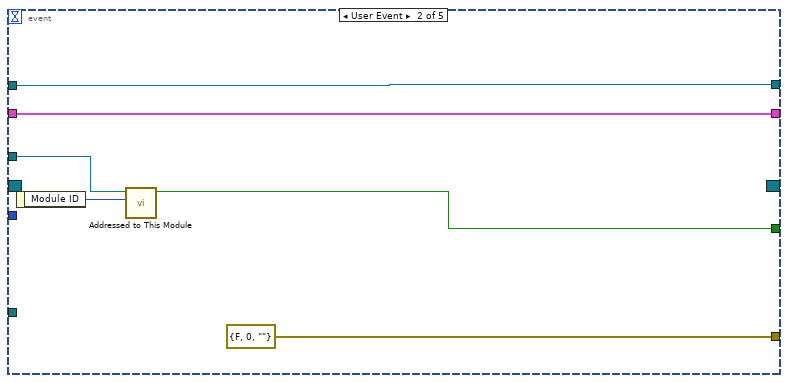
[diagram p5: hidden frame]
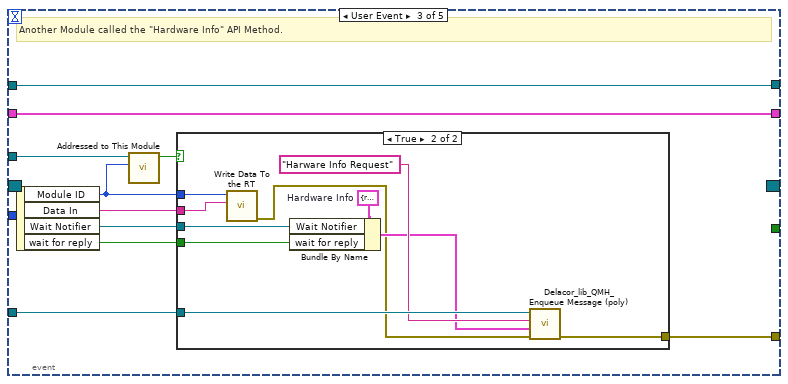
[diagram p6: hidden frame]
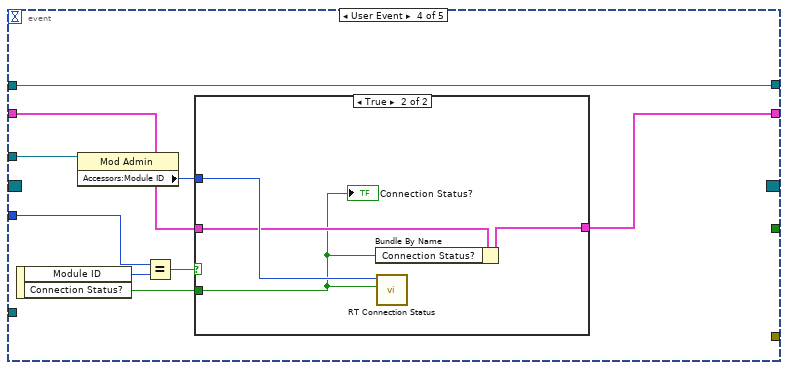
[diagram p8: hidden frame]
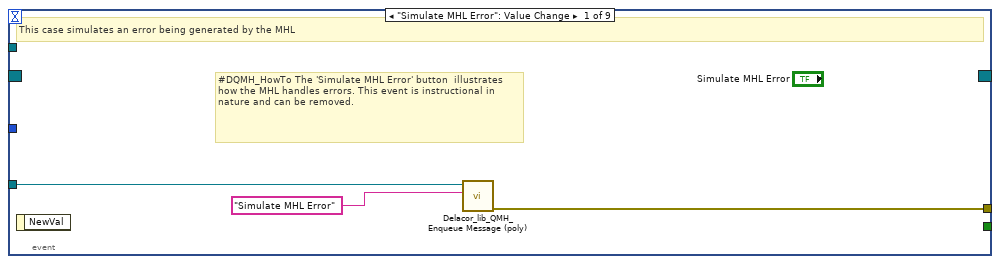
[diagram p11: hidden frame]
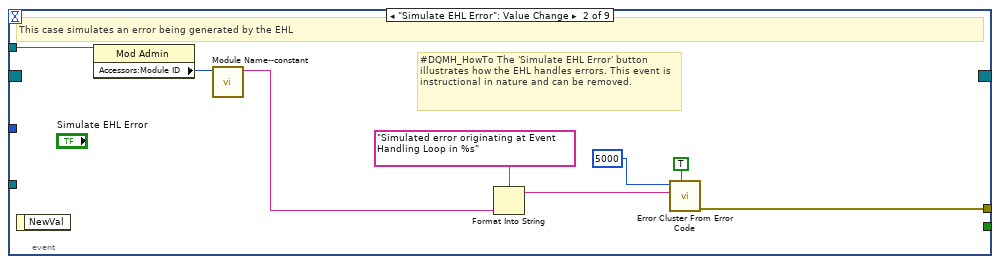
[diagram p12: hidden frame]
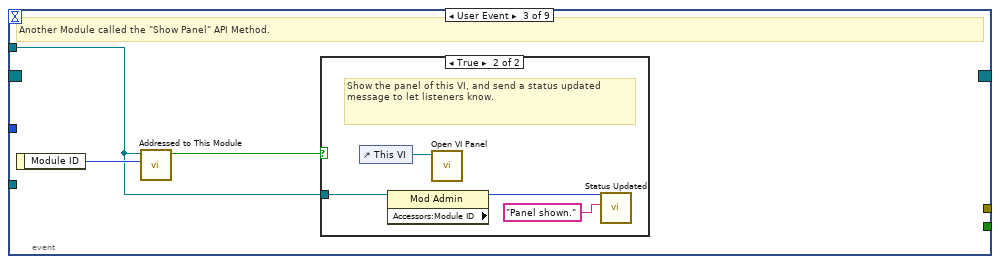
[diagram p13: hidden frame]
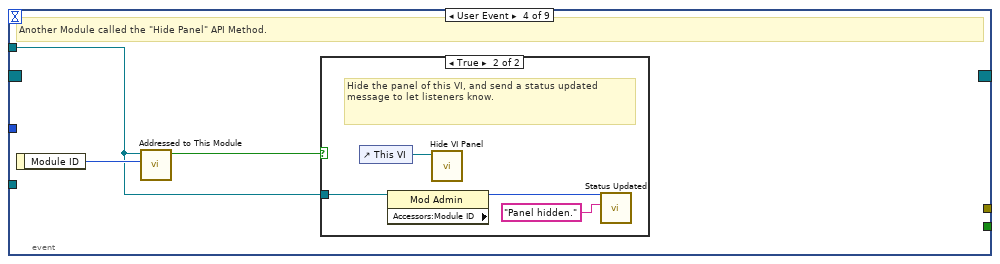
[diagram p15: hidden frame]
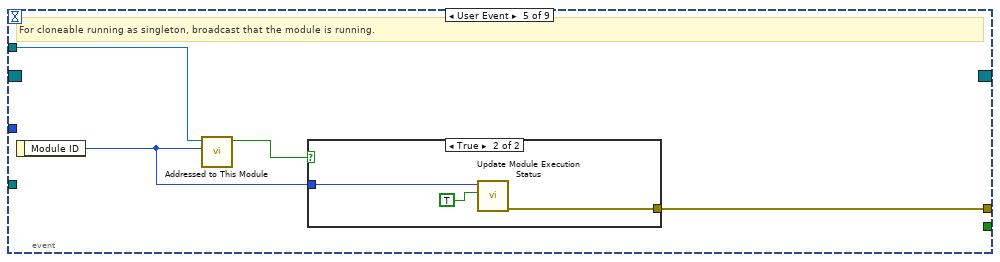
[diagram p17: hidden frame]
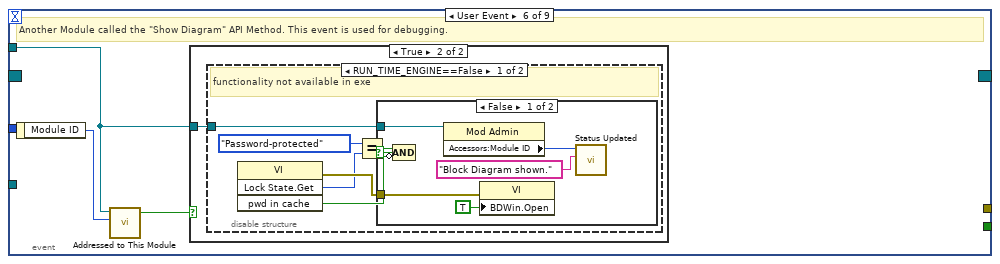
[diagram p19: hidden frame]
diagram:
  (unwired) T18 {"Serial Hardware Info JSON Format"={"Command"="", "SubCmd"="", "Channel"=[]}, "Hardware Info JSON Format"={"Command"="", "SubCmd"="", "Input"=[], "Output"=[]}, "Hardware Info JSON Format"={"Command"="", "SubCmd"="", "Input"=[], "Output"=[]}, "Ethernet IP Address JSON Format"={"Command"="", "SubCmd"="", "IP"=[]}} ("Hardware Info")
  (unwired) cluster{"AI":T6, "DI":T3, "Async":T10} {"AI"={"Interface"="AIO", "Interface Data"={"Command"="Configure", "SubCmd"="AI", "Data"=[{"Channel"="Mod2/ai0", "Min Value"=-5.0, "Max Value"=5.0, "Type"="Voltage", "Terminal Configure"=10083, "Dynamic"=0, "Dyn Type"="", "Data"=[], "File Name"="", "Column"=0, "Frequency"=0.0}, {"Channel"="Mod2/ai1", "Min Value"=-5.0, "Max Value"=5.0, "Type"="Voltage", "Terminal Configure"=10083, "Dynamic"=0, "Dyn Type"="", "Data"=[], "File Name"="", "Column"=0, "Frequency"=0.0}, {"Channel"="Mod2/ai2", "Min Value"=-5.0, "Max Value"=5.0, "Type"="Voltage", "Terminal Configure"=10083, "Dynamic"=0, "Dyn Type"="", "Data"=[], "File Name"="", "Column"=0, "Frequency"=0.0}, {"Channel"="Mod2/ai3", "Min Value"=-5.0, "Max Value"=5.0, "Type"="Voltage", "Terminal Configure"=10083, "Dynamic"=0, "Dyn Type"="", "Data"=[], "File Name"="", "Column"=0, "Frequency"=0.0}, {"Channel"="Mod2/ai4", "Min Value"=-5.0, "Max Value"=5.0, "Type"="Voltage", "Terminal Configure"=10083, "Dynamic"=0, "Dyn Type"="", "Data"=[], "File Name"="", "Column"=0, "Frequency"=0.0}, {"Channel"="Mod2/ai5", "Min Value"=-5.0, "Max Value"=5.0, "Type"="Voltage", "Terminal Configure"=10083, "Dynamic"=0, "Dyn Type"="", "Data"=[], "File Name"="", "Column"=0, "Frequency"=0.0}, {"Channel"="Mod2/ai6", "Min Value"=-5.0, "Max Value"=5.0, "Type"="Voltage", "Terminal Configure"=10083, "Dynamic"=0, "Dyn Type"="", "Data"=[], "File Name"="", "Column"=0, "Frequency"=0.0}, {"Channel"="Mod2/ai7", "Min Value"=-5.0, "Max Value"=5.0, "Type"="Voltage", "Terminal Configure"=10083, "Dynamic"=0, "Dyn Type"="", "Data"=[], "File Name"="", "Column"=0, "Frequency"=0.0}, {"Channel"="Mod2/ai8", "Min Value"=-5.0, "Max Value"=5.0, "Type"="Voltage", "Terminal Configure"=10083, "Dynamic"=0, "Dyn Type"="", "Data"=[], "File Name"="", "Column"=0, "Frequency"=0.0}, {"Channel"="Mod2/ai9", "Min Value"=-5.0, "Max Value"=5.0, "Type"="Voltage", "Terminal Configure"=10083, "Dynamic"=0, "Dyn Type"="", "Data"=[], "File Name"="", "Column"=0, "Frequency"=0.0}, {"Channel"="Mod2/ai10", "Min Value"=-5.0, "Max Value"=5.0, "Type"="Voltage", "Terminal Configure"=10083, "Dynamic"=0, "Dyn Type"="", "Data"=[], "File Name"="", "Column"=0, "Frequency"=0.0}, {"Channel"="Mod2/ai11", "Min Value"=-5.0, "Max Value"=5.0, "Type"="Voltage", "Terminal Configure"=10083, "Dynamic"=0, "Dyn Type"="", "Data"=[], "File Name"="", "Column"=0, "Frequency"=0.0}, {"Channel"="Mod2/ai12", "Min Value"=-5.0, "Max Value"=5.0, "Type"="Voltage", "Terminal Configure"=10083, "Dynamic"=0, "Dyn Type"="", "Data"=[], "File Name"="", "Column"=0, "Frequency"=0.0}, {"Channel"="Mod2/ai13", "Min Value"=-5.0, "Max Value"=5.0, "Type"="Voltage", "Terminal Configure"=10083, "Dynamic"=0, "Dyn Type"="", "Data"=[], "File Name"="", "Column"=0, "Frequency"=0.0}, {"Channel"="Mod2/ai14", "Min Value"=-5.0, "Max Value"=5.0, "Type"="Voltage", "Terminal Configure"=10083, "Dynamic"=0, "Dyn Type"="", "Data"=[], "File Name"="", "Column"=0, "Frequency"=0.0}, {"Channel"="Mod2/ai15", "Min Value"=-5.0, "Max Value"=5.0, "Type"="Voltage", "Terminal Configure"=10083, "Dynamic"=0, "Dyn Type"="", "Data"=[], "File Name"="", "Column"=0, "Frequency"=0.0}, {"Channel"="Mod2/ai16", "Min Value"=-5.0, "Max Value"=5.0, "Type"="Voltage", "Terminal Configure"=10083, "Dynamic"=0, "Dyn Type"="", "Data"=[], "File Name"="", "Column"=0, "Frequency"=0.0}, {"Channel"="Mod2/ai17", "Min Value"=-5.0, "Max Value"=5.0, "Type"="Voltage", "Terminal Configure"=10083, "Dynamic"=0, "Dyn Type"="", "Data"=[], "File Name"="", "Column"=0, "Frequency"=0.0}, {"Channel"="Mod2/ai18", "Min Value"=-5.0, "Max Value"=5.0, "Type"="Voltage", "Terminal Configure"=10083, "Dynamic"=0, "Dyn Type"="", "Data"=[], "File Name"="", "Column"=0, "Frequency"=0.0}, {"Channel"="Mod2/ai19", "Min Value"=-5.0, "Max Value"=5.0, "Type"="Voltage", "Terminal Configure"=10083, "Dynamic"=0, "Dyn Type"="", "Data"=[], "File Name"="", "Column"=0, "Frequency"=0.0}, {"Channel"="Mod2/ai20", "Min Value"=-5.0, "Max Value"=5.0, "Type"="Voltage", "Terminal Configure"=10083, "Dynamic"=0, "Dyn Type"="", "Data"=[], "File Name"="", "Column"=0, "Frequency"=0.0}, {"Channel"="Mod2/ai21", "Min Value"=-5.0, "Max Value"=5.0, "Type"="Voltage", "Terminal Configure"=10083, "Dynamic"=0, "Dyn Type"="", "Data"=[], "File Name"="", "Column"=0, "Frequency"=0.0}, {"Channel"="Mod2/ai22", "Min Value"=-5.0, "Max Value"=5.0, "Type"="Voltage", "Terminal Configure"=10083, "Dynamic"=0, "Dyn Type"="", "Data"=[], "File Name"="", "Column"=0, "Frequency"=0.0}, {"Channel"="Mod2/ai23", "Min Value"=-5.0, "Max Value"=5.0, "Type"="Voltage", "Terminal Configure"=10083, "Dynamic"=0, "Dyn Type"="", "Data"=[], "File Name"="", "Column"=0, "Frequency"=0.0}, {"Channel"="Mod2/ai24", "Min Value"=-5.0, "Max Value"=5.0, "Type"="Voltage", "Terminal Configure"=10083, "Dynamic"=0, "Dyn Type"="", "Data"=[], "File Name"="", "Column"=0, "Frequency"=0.0}, {"Channel"="Mod2/ai25", "Min Value"=-5.0, "Max Value"=5.0, "Type"="Voltage", "Terminal Configure"=10083, "Dynamic"=0, "Dyn Type"="", "Data"=[], "File Name"="", "Column"=0, "Frequency"=0.0}, {"Channel"="Mod2/ai26", "Min Value"=-5.0, "Max Value"=5.0, "Type"="Voltage", "Terminal Configure"=10083, "Dynamic"=0, "Dyn Type"="", "Data"=[], "File Name"="", "Column"=0, "Frequency"=0.0}, {"Channel"="Mod2/ai27", "Min Value"=-5.0, "Max Value"=5.0, "Type"="Voltage", "Terminal Configure"=10083, "Dynamic"=0, "Dyn Type"="", "Data"=[], "File Name"="", "Column"=0, "Frequency"=0.0}, {"Channel"="Mod2/ai28", "Min Value"=-5.0, "Max Value"=5.0, "Type"="Voltage", "Terminal Configure"=10083, "Dynamic"=0, "Dyn Type"="", "Data"=[], "File Name"="", "Column"=0, "Frequency"=0.0}, {"Channel"="Mod2/ai29", "Min Value"=-5.0, "Max Value"=5.0, "Type"="Voltage", "Terminal Configure"=10083, "Dynamic"=0, "Dyn Type"="", "Data"=[], "File Name"="", "Column"=0, "Frequency"=0.0}, {"Channel"="Mod2/ai30", "Min Value"=-5.0, "Max Value"=5.0, "Type"="Voltage", "Terminal Configure"=10083, "Dynamic"=0, "Dyn Type"="", "Data"=[], "File Name"="", "Column"=0, "Frequency"=0.0}, {"Channel"="Mod2/ai31", "Min Value"=-5.0, "Max Value"=5.0, "Type"="Voltage", "Terminal Configure"=65535, "Dynamic"=0, "Dyn Type"="", "Data"=[], "File Name"="", "Column"=0, "Frequency"=0.0}], "Timing"={"samples per channel"=4, "sample mode"=10123, "Sampling Rate"=2.0}}}, "DI"={"Interface"="DIO", "Interface Data"={"Command"="Configure", "SubCmd"="DI", "Frequency"=500, "Data"=[{"Channel"="Mod3/port0/line0", "Data"=[0], "Identification Name"=""}, {"Channel"="Mod3/port0/line1", "Data"=[0], "Identification Name"=""}, {"Channel"="Mod3/port0/line2", "Data"=[0], "Identification Name"=""}, {"Channel"="Mod3/port0/line3", "Data"=[0], "Identification Name"=""}, {"Channel"="Mod3/port0/line4", "Data"=[0], "Identification Name"=""}, {"Channel"="Mod3/port0/line5", "Data"=[0], "Identification Name"=""}, {"Channel"="Mod3/port0/line6", "Data"=[0], "Identification Name"=""}, {"Channel"="Mod3/port0/line7", "Data"=[0], "Identification Name"=""}, {"Channel"="Mod3/port0/line8", "Data"=[0], "Identification Name"=""}, {"Channel"="Mod3/port0/line9", "Data"=[0], "Identification Name"=""}, {"Channel"="Mod3/port0/line10", "Data"=[0], "Identification Name"=""}, {"Channel"="Mod3/port0/line11", "Data"=[0], "Identification Name"=""}, {"Channel"="Mod3/port0/line12", "Data"=[0], "Identification Name"=""}, {"Channel"="Mod3/port0/line13", "Data"=[0], "Identification Name"=""}, {"Channel"="Mod3/port0/line14", "Data"=[0], "Identification Name"=""}, {"Channel"="Mod3/port0/line15", "Data"=[0], "Identification Name"=""}, {"Channel"="Mod3/port0/line16", "Data"=[0], "Identification Name"=""}, {"Channel"="Mod3/port0/line17", "Data"=[0], "Identification Name"=""}, {"Channel"="Mod3/port0/line18", "Data"=[0], "Identification Name"=""}, {"Channel"="Mod3/port0/line19", "Data"=[0], "Identification Name"=""}, {"Channel"="Mod3/port0/line20", "Data"=[0], "Identification Name"=""}, {"Channel"="Mod3/port0/line21", "Data"=[0], "Identification Name"=""}, {"Channel"="Mod3/port0/line22", "Data"=[0], "Identification Name"=""}, {"Channel"="Mod3/port0/line23", "Data"=[0], "Identification Name"=""}, {"Channel"="Mod3/port0/line24", "Data"=[0], "Identification Name"=""}, {"Channel"="Mod3/port0/line25", "Data"=[0], "Identification Name"=""}, {"Channel"="Mod3/port0/line26", "Data"=[0], "Identification Name"=""}, {"Channel"="Mod3/port0/line27", "Data"=[0], "Identification Name"=""}, {"Channel"="Mod3/port0/line28", "Data"=[0], "Identification Name"=""}, {"Channel"="Mod3/port0/line29", "Data"=[0], "Identification Name"=""}, {"Channel"="Mod3/port0/line30", "Data"=[0], "Identification Name"=""}, {"Channel"="Mod3/port0/line31", "Data"=[0], "Identification Name"=""}, {"Channel"="Mod4/port0/line0", "Data"=[0], "Identification Name"=""}, {"Channel"="Mod4/port0/line1", "Data"=[0], "Identification Name"=""}, {"Channel"="Mod4/port0/line2", "Data"=[0], "Identification Name"=""}, {"Channel"="Mod4/port0/line3", "Data"=[0], "Identification Name"=""}, {"Channel"="Mod4/port0/line4", "Data"=[0], "Identification Name"=""}, {"Channel"="Mod4/port0/line5", "Data"=[0], "Identification Name"=""}, {"Channel"="Mod4/port0/line6", "Data"=[0], "Identification Name"=""}, {"Channel"="Mod4/port0/line7", "Data"=[0], "Identification Name"=""}, {"Channel"="Mod4/port0/line8", "Data"=[0], "Identification Name"=""}, {"Channel"="Mod4/port0/line9", "Data"=[0], "Identification Name"=""}, {"Channel"="Mod4/port0/line10", "Data"=[0], "Identification Name"=""}, {"Channel"="Mod4/port0/line11", "Data"=[0], "Identification Name"=""}, {"Channel"="Mod4/port0/line12", "Data"=[0], "Identification Name"=""}, {"Channel"="Mod4/port0/line13", "Data"=[0], "Identification Name"=""}, {"Channel"="Mod4/port0/line14", "Data"=[0], "Identification Name"=""}, {"Channel"="Mod4/port0/line15", "Data"=[0], "Identification Name"=""}, {"Channel"="Mod4/port0/line16", "Data"=[0], "Identification Name"=""}, {"Channel"="Mod4/port0/line17", "Data"=[0], "Identification Name"=""}, {"Channel"="Mod4/port0/line18", "Data"=[0], "Identification Name"=""}, {"Channel"="Mod4/port0/line19", "Data"=[0], "Identification Name"=""}, {"Channel"="Mod4/port0/line20", "Data"=[0], "Identification Name"=""}, {"Channel"="Mod4/port0/line21", "Data"=[0], "Identification Name"=""}, {"Channel"="Mod4/port0/line22", "Data"=[0], "Identification Name"=""}, {"Channel"="Mod4/port0/line23", "Data"=[0], "Identification Name"=""}, {"Channel"="Mod4/port0/line24", "Data"=[0], "Identification Name"=""}, {"Channel"="Mod4/port0/line25", "Data"=[0], "Identification Name"=""}, {"Channel"="Mod4/port0/line26", "Data"=[0], "Identification Name"=""}, {"Channel"="Mod4/port0/line27", "Data"=[0], "Identification Name"=""}, {"Channel"="Mod4/port0/line28", "Data"=[0], "Identification Name"=""}, {"Channel"="Mod4/port0/line29", "Data"=[0], "Identification Name"=""}, {"Channel"="Mod4/port0/line30", "Data"=[0], "Identification Name"=""}, {"Channel"="Mod4/port0/line31", "Data"=[0], "Identification Name"=""}]}}, "Async"={"Interface"="Async", "Interface Data"={"Command"="Configure", "SubCmd"="Async", "Data"=[{"Port"="com10", "Minor Frame Freq"=200, "Minor Frame Count"=1, "Frame Info"=[{"Frame ID"=1, "Message Info"=[{"Message"=[1], "Message Name"="m1"}]}], "Sensor Type"=0, "OIM Address"=0}]}}} ("Channel Data 2")
  # "#DQMH_HowTo This is the top-level VI of a DQMH Cloneable module. See the following video for a discussion of cloneable-specific functionality: https://bit.ly/DQMHCloneableMainWalkthrough"
  # "Note: Do not modify or remove the \"DQMH\" labels on objects. These labels are used by the Tools > DQMH Consortium > DQMH utilities."
  # "Updating the Module Admin to ensure this module can run as a stand alone next time."
  n1 = disable-structure shown="Disabled" {
    frame Disabled {
      n2 = call "TCP-Open Connection.vi"() -> ()  [unwired: 11 in, 1 out]
      n3 = call "Read TCP Data.vi"() -> ()  [unwired: 11 in, 1 out]
      n4 = call "TCP-Write.vi"() -> ()  [unwired: 11 in, 1 out]
      n5 = call "TCP-Close Connection.vi"() -> ()  [unwired: 11 in, 1 out]
    }
    frame Enabled {
    }
  }
  n6 = call "Init Module.vi"("Cloneable Module Admin in"="Module Admin") -> ("error out"=w3:errorcluster, "RT Acquisition Engine Request Events"=w2:T19, "Cloneable Module Admin out"=w7:refnum<class "Delacor_lib_QMH_Cloneable Module Admin.lvclass">)  [unwired: 8 in]
  n7 = register-events "DQMH_REG_EVENTS"(w2) -> (reference out=w10:refnum<event-registration>, error out=w1:errorcluster)  [unwired: 2 in]
  n8 = call <vilib>:"Delacor_lib_QMH_Create Message Queue.vi"("error in"=w3) -> ("error out"=w13:errorcluster, "Message Queue"=w9:refnum<class "Delacor_lib_QMH_Message Queue.lvclass">)  [unwired: 9 in]
  n9 = Merge Errors(w13, w1) -> (w12:errorcluster)
  n10 = case shown="No Error" w12 {
    selector: w12 -> [w38 w445]
    tunnel: [w40 w444] -> w16
    tunnel: [w37 w443] -> w11
    tunnel: w10 -> [w36 w443]
    tunnel: w9 -> [w35 w436]
    tunnel: [w39 _] -> w17
    tunnel: w7 -> [w34 w439]
    tunnel: [w33 _] -> w5
    tunnel: w2 -> [w32 _]
    frame No Error {
      w19 = T27 {"Status"="", "This Module ID"=-1, "RT-IP"="", "Hardware Info Request Ref"={"Wait Notifier"=refnum, "wait for reply"=FALSE}, "RT-Data's"={"DO Info"={"Channels"=[], "Data"=[], "Time"=""}, "AI-Data From RT--Cluster"={"Channel Name's"=[], "Channel Data's"=[], "Date & Time"=""}, "Hardware Information"=variant(cluster{"Serial Hardware Info JSON Format":cluster{"Command":string, "SubCmd":string, "Channel":string[]}, "Analog HW Info JSON Format":cluster{"Command":string, "SubCmd":string, "Input":string[], "Output":string[]}, "Digital HW Info JSON Format":cluster{"Command":string, "SubCmd":string, "Input":string[], "Output":string[]}, "Ethernet IP Address JSON Format":cluster{"Command":string, "SubCmd":string, "IP":string[]}} {"Serial Hardware Info JSON Format"={"Command"="", "SubCmd"="", "Channel"=[]}, "Analog HW Info JSON Format"={"Command"="", "SubCmd"="", "Input"=[], "Output"=[]}, "Digital HW Info JSON Format"={"Command"="", "SubCmd"="", "Input"=[], "Output"=[]}, "Ethernet IP Address JSON Format"={"Command"="", "SubCmd"="", "IP"=[]}})}, "Connection Status?"=FALSE} ("Data Cluster")
      n11 = call "Start Module.vi"() -> ("error out"=w24:errorcluster, "Wait for Event Sync?"=w22:bool, "TCP-IP Engine Broadcast Events"=w25:T30, "Module ID"=w21:i32)  [unwired: 8 in]
      n12 = register-events ("DQMH_HELPER_REGFOREVENTS")(error in=w24, w32, w25) -> (reference out=w30:refnum<event-registration>, error out=w23:errorcluster)  [unwired: 1 in]
      n13 = call "Synchronize Module Events.vi"("error in"=w23, "Wait for Event Sync?"=w22, "Module ID in"=w21) -> ("Module ID out"=w20:i32)  [unwired: 7 in, 1 out]
      "TCP-IP Module ID" <- w20
      n14 = call <vilib>:"Init Helper Loop Info-v2.vi"() -> ("Helper Loop Periodic Timing"=w29:refnum<class "Helper Loop Periodic Timing.lvclass">)  [unwired: 1 in]
      n15 = while {
        tunnel: w35 -> [w117]
        shift-right: [w120] -> w37
        shift-left: w36 -> [w121]
        tunnel: [w122] -> w39
        tunnel: w34 -> [w118]
        tunnel: w20 -> [w116]
        stop <- w119 stop-if-true
        # "Event Handling Loop"
        n16 = event "DQMH_EVENT_MAIN" shown="[8] <RT Acquisition Engine Request Events.Write Data To the RT>: User Event" {
          selector: w121 -> [_ _ _ _ _ _ _ _ _]
          dyn-events: [_ _ _ _ _ _ _ _ _] -> w120
          timeout: _ -> [_ _ _ _ _ _ _ _ _]
          tunnel: [_ _ _ _ _ _ w175 _ _] -> w119
          tunnel: w117 -> [w125 _ _ _ _ _ w178 w197 w217]
          tunnel: [w126 w134 _ _ w152 _ w179 w200 w211] -> w123
          tunnel: w118 -> [_ w133 w135 w142 w150 w156 w177 w198 w215]
          tunnel: w116 -> [_ _ _ _ _ _ _ _ _]
          event "Simulate MHL Error": Value Change {
            # "#DQMH_HowTo The 'Simulate MHL Error' button  illustrates how the MHL handles errors. This event is instructional in nature and can be removed."
            # "This case simulates an error being generated by the MHL"
            n17 = event-data() -> ()  [unwired: 1 in, 1 out]
            n18 = call-poly <vilib>:"Delacor_lib_QMH_Enqueue Message (poly).vi"("Message"="Simulate MHL Error", "Message Queue in"=w125) -> ("error out"=w126:errorcluster)  [unwired: 8 in, 1 out]
          }
          event "Simulate EHL Error": Value Change {
            # "#DQMH_HowTo The 'Simulate EHL Error' button  illustrates how the EHL handles errors. This event is instructional in nature and can be removed."
            # "This case simulates an error being generated by the EHL"
            n19 = event-data() -> ()  [unwired: 1 in, 1 out]
            n20 = property on="Property Node" class="Mod Admin"(reference=w133) -> ("Accessors:Module ID"=w132:i32)  [unwired: 1 in, 2 out]
            n21 = call "Module Name--constant.vi"("Module ID"=w132) -> ("Module Name"=w127:string)  [unwired: 10 in]
            n22 = Format Into String(format string="Simulated error originating at Event Handling Loop in %s", w127) -> (resulting string=w130:string)  [unwired: 2 in, 1 out]
            n23 = call <vilib>:"Error Cluster From Error Code.vi"("show call chain? (False)"=TRUE, "error message (\"\")"=w130, "error code (0)"=5000) -> ("error out"=w134:errorcluster)  [unwired: 6 in]
          }
          event User Event {
            # "Another Module called the \"Show Panel\" API Method."
            n24 = event-data() -> ("Module ID"=w136:i32)  [unwired: 1 in]
            n25 = call "Addressed to This Module.vi"("Module ID from Argument"=w136, "Module Admin"=w135) -> ("Addressed to this instance?"=w137:bool)  [unwired: 8 in, 1 out]
            n26 = case shown="True" w137 {
              tunnel: w135 -> [_ w139]
              frame False {
              }
              frame True {
                # "Show the panel of this VI, and send a status updated message to let listeners know."
                n27 = control-ref of="This VI"() -> (w141:refnum<vi>)
                n28 = property on="Property Node" class="Mod Admin"(reference=w139) -> ("Accessors:Module ID"=w138:i32)  [unwired: 1 in, 2 out]
                n29 = call "Open VI Panel.vi"("VI"=w141) -> ()  [unwired: 10 in, 1 out]
                n30 = call "Status Updated.vi"("Status"="Panel shown." ("format string"), "Module ID"=w138) -> ()  [unwired: 9 in, 1 out]
              }
            }
          }
          event User Event {
            # "Another Module called the \"Hide Panel\" API Method."
            n31 = event-data() -> ("Module ID"=w143:i32)  [unwired: 1 in]
            n32 = call "Addressed to This Module.vi"("Module ID from Argument"=w143, "Module Admin"=w142) -> ("Addressed to this instance?"=w144:bool)  [unwired: 8 in, 1 out]
            n33 = case shown="True" w144 {
              tunnel: w142 -> [_ w146]
              frame False {
              }
              frame True {
                # "Hide the panel of this VI, and send a status updated message to let listeners know."
                n34 = control-ref of="This VI"() -> (w148:refnum<vi>)
                n35 = property on="Property Node" class="Mod Admin"(reference=w146) -> ("Accessors:Module ID"=w145:i32)  [unwired: 1 in, 2 out]
                n36 = call "Hide VI Panel.vi"("VI"=w148) -> ()  [unwired: 10 in, 1 out]
                n37 = call "Status Updated.vi"("Status"="Panel hidden." ("format string"), "Module ID"=w145) -> ()  [unwired: 9 in, 1 out]
              }
            }
          }
          event User Event {
            # "For cloneable running as singleton, broadcast that the module is running."
            n38 = event-data() -> ("Module ID"=w149:i32)  [unwired: 1 in]
            n39 = call "Addressed to This Module.vi"("Module ID from Argument"=w149, "Module Admin"=w150) -> ("Addressed to this instance?"=w151:bool)  [unwired: 8 in, 1 out]
            n40 = case shown="True" w151 {
              tunnel: [_ w155] -> w152
              tunnel: w149 -> [_ w154]
              frame False {
              }
              frame True {
                n41 = call "Update Module Execution Status.vi"("Running?"=TRUE, "Module ID"=w154) -> ("error out"=w155:errorcluster)  [unwired: 9 in]
              }
            }
          }
          event User Event {
            # "Another Module called the \"Show Diagram\" API Method. This event is used for debugging."
            n42 = event-data() -> ("Module ID"=w157:i32)  [unwired: 1 in]
            n43 = call "Addressed to This Module.vi"("Module ID from Argument"=w157, "Module Admin"=w156) -> ("Addressed to this instance?"=w158:bool)  [unwired: 8 in, 1 out]
            n44 = case shown="True" w158 {
              tunnel: w156 -> [_ w159]
              frame False {
              }
              frame True {
                n45 = disable-structure shown="RUN_TIME_ENGINE==False" {
                  disable-tunnel: w159 -> [w160 _]
                  frame condition #0 (active) {
                    # "functionality not available in exe"
                    n46 = invoke on="Invoke Node" class="VI" method="Lock State.Get"() -> (error out=w166:errorcluster, "Get Lock State"=w165:T21, "pwd in cache"=w162:bool)  [unwired: 4 in, 1 out]
                    n47 = Equal?(x=T21."Password-protected", y=w165) -> (x = y?=w163:bool)
                    n48 = Compound Arithmetic op=AND(w163, invert w162) -> (w161:bool)
                    n49 = case shown="False" w161 {
                      tunnel: w166 -> [w171 _]
                      tunnel: w160 -> [w168 _]
                      frame False {
                        n50 = property on="Property Node" class="Mod Admin"(reference=w168) -> ("Accessors:Module ID"=w167:i32)  [unwired: 1 in, 2 out]
                        n51 = property on="Property Node" class="VI"(error in=w171, "BDWin.Open"=TRUE ("Block Diagram Window:Open")) -> ()  [unwired: 1 in, 2 out]
                        n52 = call "Status Updated.vi"("Status"="Block Diagram shown." ("format string"), "Module ID"=w167) -> ()  [unwired: 9 in, 1 out]
                      }
                      frame True {
                        # "Password-protected VI, and the password is not in the cache. Do not show the diagram."
                      }
                    }
                  }
                  frame condition #1 {
                  }
                }
              }
            }
          }
          event User Event {
            # "Another Module called the \"Stop Module\" API Method  or the Message Handling Loop below."
            n53 = event-data() -> ("Module ID"=w173:i32, "Wait for Module to stop?"=w174:bool, "Origin"=w172:string)  [unwired: 1 in]
            n54 = call "Addressed to This Module.vi"("Module ID from Argument"=w173, "Module Admin"=w177) -> ("Addressed to this instance?"=w176:bool)  [unwired: 8 in, 1 out]
            n55 = case shown="True" w176 {
              tunnel: [_ w193] -> w179
              tunnel: w178 -> [_ w182]
              tunnel: [_ TRUE] -> w175
              tunnel: w174 -> [_ w185]
              tunnel: w173 -> [_ w187]
              tunnel: w172 -> [_ w183]
              frame False {
              }
              frame True {
                # "The event can get fired from the Exit message. The queue gets destroyed there. In this case, the Enqueue VI will return error 1. It is safe to ignore, because the module is already exiting."
                n56 = local write "Status"(w183) -> ()
                n57 = Bundle By Name(cluster=T22 {"Module ID"=-1, "Origin"="", "Exit via Stop Module Req?"=FALSE, "Wait for Module to stop?"=FALSE} ("Stop Argument"), "Module ID"=w187, "Exit via Stop Module Req?"=TRUE, "Wait for Module to stop?"=w185) -> (w184:T22)
                n58 = call-dynamic "Delacor_lib_QMH_Flush Messages.vi"("Message Queue in"=w182) -> ("error out"=w180:errorcluster, "Message Queue out"=w181:refnum<class "Delacor_lib_QMH_Message Queue.lvclass">)  [unwired: 7 in, 2 out]
                n59 = call-poly <vilib>:"Delacor_lib_QMH_Enqueue Message (poly).vi"("Priority Message? (F)"=TRUE, "error in"=w180, "Message Data"=w184, "Message"="Exit", "Message Queue in"=w181) -> ("error out"=w194:errorcluster)  [unwired: 5 in, 1 out]
                n60 = call <vilib>:"Clear Errors.vi"("error in (no error)"=w194, "specific error code to clear (0: all)"=1) -> ("error out"=w193:errorcluster)  [unwired: 4 in, 1 out]
              }
            }
          }
          event Panel Close? {
            w199 = TRUE  # Discard the event, the MHL is responsible for closing and stopping this VI.
            # "Hide the panel or send the 'Exit' message if the user clicks the 'X' on the module main VI panel."
            n61 = event-data() -> ()  [unwired: 1 in, 1 out]
            n62 = property on="Property Node" class="Mod Admin"(reference=w198) -> (reference out=w195:refnum<class "Delacor_lib_QMH_Cloneable Module Admin.lvclass">, "Accessors:External Launch"=w196:bool)  [unwired: 1 in, 1 out]
            n63 = case shown="True" w196 {
              tunnel: w197 -> [_ w208]
              tunnel: [_ w209] -> w200
              tunnel: w195 -> [w203 _]
              frame True {
                # "If externally launched, clicking the 'X' hides the panel, but doesn't close it."
                n64 = property on="Property Node" class="Mod Admin"(reference=w203) -> ("Accessors:Module ID"=w202:i32)  [unwired: 1 in, 2 out]
                n65 = call "Status Updated.vi"("Status"="Panel hidden." ("format string"), "Module ID"=w202) -> ("error out"=w201:errorcluster)  [unwired: 9 in]
                n66 = control-ref of="This VI"() -> (w205:refnum<vi>)
                n67 = call "Hide VI Panel.vi"("error in"=w201, "VI"=w205) -> ()  [unwired: 9 in, 1 out]
              }
              frame False {
                # "If run as a stand-alone VI, clicking the panel 'X' stops the VI."
                n68 = call-poly <vilib>:"Delacor_lib_QMH_Enqueue Message (poly).vi"("Priority Message? (F)"=TRUE, "Message"="Exit", "Message Queue in"=w208) -> ("error out"=w209:errorcluster)  [unwired: 7 in, 1 out]
              }
            }
            n69 = event-data ("Event Filter Node")("Discard?"=w199) -> ()  [unwired: 1 in, 1 out]
          }
          event User Event {
            # "Another Module called the \"Write Data To the RT\" API Method."
            n70 = event-data() -> ("Module ID"=w210:i32, "Data In"=w212:string)  [unwired: 1 in]
            n71 = Bundle(cluster=T23 {"Module ID"=-1, "Data In"=""} ("Write Data To the RT Argument"), "Module ID"=w210, "Data In"=w212) -> (w213:T23)
            n72 = call "Addressed to This Module.vi"("Module ID from Argument"=w210, "Module Admin"=w215) -> ("Addressed to this instance?"=w216:bool)  [unwired: 8 in, 1 out]
            n73 = case shown="True" w216 {
              tunnel: w217 -> [_ w222]
              tunnel: w213 -> [_ w220]
              tunnel: [_ w219] -> w211
              frame False {
              }
              frame True {
                n74 = call-poly <vilib>:"Delacor_lib_QMH_Enqueue Message (poly).vi"("Priority Message? (F)"=TRUE, "Message Data"=w220, "Message"="Write Data To the RT", "Message Queue in"=w222) -> ("error out"=w219:errorcluster)  [unwired: 6 in, 1 out]
              }
            }
          }
        }
        n75 = call-dynamic "Delacor_lib_QMH_Error Handler - Event Handling Loop.vi"("error in"=w123, "Message Queue in"=w117) -> ("dup error in"=w122:errorcluster)  [unwired: 8 in, 1 out]
      }
      n76 = call <vilib>:"Set Helper Loop Period.vi"("Period (ms)"=100, "Helper Loop Periodic Timing in"=w29) -> ("Helper Loop Periodic Timing out"=w28:refnum<class "Helper Loop Periodic Timing.lvclass">)  [unwired: 13 in]
      n77 = while "DQMH_HELPER_LOOP" {
        shift-right: [w53] -> w27
        shift-left: w28 -> [w43]
        shift-right: [w51] -> w31
        shift-left: w30 -> [w52]
        tunnel: w35 -> [w48]
        tunnel: w34 -> [w46]
        tunnel: w20 -> [w45]
        shift-right: [w41] -> _
        shift-left: w19 -> [w42]
        stop <- w50 stop-if-true
        w47 = "TCP-IP Read"  # DQMH_HELPER_LOOP_NAME
        # "TCP-IP Read"
        n78 = call <vilib>:"Get Timeout.vi"("Helper Loop Periodic Timing"=w43) -> ("Timeout (ms)"=w44:i32)  [unwired: 12 in, 2 out]
        n79 = event "DQMH_HELPER_EVENT_STRUCTURE" shown="[4] <TCP-IP Engine Broadcast Events.TCP-Read Data Out>: User Event" {
          selector: w52 -> [_ _ _ _ _]
          dyn-events: [_ _ _ _ _] -> w51
          timeout: w44 -> [_ _ _ _ _]
          tunnel: w43 -> [w57 w69 w79 w98 w111]
          tunnel: [w56 w69 w79 w98 w111] -> w53
          tunnel: [_ w66 _ _ _] -> w50
          tunnel: [_ errorcluster {"status"=FALSE, "code"=0, "source"=""} ("error constant") w71 _ w109] -> w49
          tunnel: w48 -> [_ _ w72 _ w105]
          tunnel: w46 -> [_ w67 w75 w95 _]
          tunnel: w45 -> [w59 _ _ w97 w106]
          tunnel: w42 -> [w55 w64 w70 w93 w104]
          tunnel: [w55 w64 w70 w92 w104] -> w41
          event Timeout {
            n80 = event-data() -> ("Time"=w58:u32)  [unwired: 1 in]
            n81 = Unbundle By Name(w55) -> ("Connection Status?"=w54:bool)
            n82 = call <vilib>:"Update Last Execution Time-v2.vi"("Time"=w58, "Helper Loop Periodic Timing in"=w57) -> ("Helper Loop Periodic Timing out"=w56:refnum<class "Helper Loop Periodic Timing.lvclass">)  [unwired: 12 in, 1 out]
            n83 = case shown="True" w54 {
              tunnel: w59 -> [_ w60]
              frame False {
              }
              frame True {
                n84 = call "Read TCP Data.vi"("bytes to read"=4, "timeout ms (25000)"=500, "mode (standard)"=T20."Buffered", "Module ID"=w60) -> ()  [unwired: 7 in, 1 out]
              }
            }
          }
          event User Event {
            n85 = event-data() -> ("Module ID"=w65:i32)  [unwired: 1 in]
            n86 = call "Addressed to This Module.vi"("Module ID from Argument"=w65, "Module Admin"=w67) -> ("Addressed to this instance?"=w66:bool)  [unwired: 8 in, 1 out]
          }
          event User Event {
            # "Another Module called the \"Hardware Info\" API Method."
            n87 = event-data() -> ("Module ID"=w74:i32, "Data In"=w73:string, "Wait Notifier"=w77:refnum<notifier>, "wait for reply"=w76:bool)  [unwired: 1 in]
            n88 = call "Addressed to This Module.vi"("Module ID from Argument"=w74, "Module Admin"=w75) -> ("Addressed to this instance?"=w78:bool)  [unwired: 8 in, 1 out]
            n89 = case shown="True" w78 {
              tunnel: w77 -> [_ w84]
              tunnel: w76 -> [_ w83]
              tunnel: w74 -> [_ w89]
              tunnel: w73 -> [_ w88]
              tunnel: w72 -> [_ w87]
              tunnel: [_ w81] -> w71
              frame False {
              }
              frame True {
                w85 = T31 {"Wait Notifier"=refnum, "wait for reply"=FALSE}  # Hardware Info
                n90 = call "Write Data To the RT.vi"("Data In"=w88, "Module ID"=w89) -> ("error out"=w80:errorcluster)  [unwired: 9 in]
                n91 = Bundle By Name(cluster=w85, "Wait Notifier"=w84, "wait for reply"=w83) -> (w82:T31)
                n92 = call-poly <vilib>:"Delacor_lib_QMH_Enqueue Message (poly).vi"("error in"=w80, "Message Data"=w82, "Message"="Harware Info Request", "Message Queue in"=w87) -> ("error out"=w81:errorcluster)  [unwired: 6 in, 1 out]
              }
            }
          }
          event User Event {
            n93 = event-data() -> ("Module ID"=w96:i32, "Connection Status?"=w91:bool)  [unwired: 1 in]
            n94 = property class="Mod Admin"(reference=w95) -> ("Accessors:Module ID"=w94:i32)  [unwired: 1 in, 2 out]
            n95 = Equal?(x=w97, y=w96) -> (x = y?=w90:bool)
            n96 = case shown="True" w90 {
              tunnel: w94 -> [_ w103]
              tunnel: w93 -> [w99 w102]
              tunnel: [w99 w101] -> w92
              tunnel: w91 -> [_ w100]
              frame False {
              }
              frame True {
                n97 = Bundle By Name(cluster=w102, "Connection Status?"=w100) -> (w101:T27)
                n98 = call "RT Connection Status.vi"("RT Connection Status?"=w100, "Module ID"=w103) -> ()  [unwired: 9 in, 1 out]
                "Connection Status?" <- w100
              }
            }
          }
          event User Event {
            n99 = event-data() -> ("Module ID"=w108:i32, "TCP-IP Data Out"=w107:string)  [unwired: 1 in]
            n100 = Equal?(x=w106, y=w108) -> (x = y?=w110:bool)
            n101 = case shown="True" w110 {
              tunnel: w105 -> [_ w114]
              tunnel: [_ w113] -> w109
              tunnel: w107 -> [_ w112]
              frame False {
              }
              frame True {
                n102 = call-poly <vilib>:"Delacor_lib_QMH_Enqueue Message (poly).vi"("Message Data"=w112, "Message"="Decode TCP-Data", "Message Queue in"=w114) -> ("error out"=w113:errorcluster)  [unwired: 7 in, 1 out]
                "TCP-IP Data Out 2" <- w112
              }
            }
          }
        }
        n103 = call-dynamic "Delacor_lib_QMH_Error Handler - Helper Loop.vi"("Error Debug"=w47, "error in"=w49, "Message Queue in"=w48) -> ()  [unwired: 7 in, 2 out]
      }
      n104 = while {
        tunnel: w35 -> [w224]
        shift-right: [w231] -> _
        shift-left: w19 -> [w232]
        tunnel: w38 -> [w235]
        tunnel: [w233] -> w40
        tunnel: w34 -> [w226]
        tunnel: [w225] -> w33
        tunnel: w20 -> [w223]
        stop <- w230 stop-if-true
        # "Message Handling Loop"
        n105 = call-dynamic "Delacor_lib_QMH_Dequeue Message.vi"("error in"=w235, "Message Queue in"=w224) -> ("error out"=w234:errorcluster, "Message Data"=w228:variant, "Message"=w229:string, "Message Queue out"=w227:refnum<class "Delacor_lib_QMH_Message Queue.lvclass">)  [unwired: 6 in]
        n106 = case "DQMH_MESSAGE_CASES" shown="\"Decode TCP-Data\"" w229 {
          selector: w229 -> [_ _ _ _ _ _ _ _ _ _ _ _ _ _ _ _ _ w425]
          tunnel: w227 -> [w241 w263 _ _ _ _ _ _ _ _ w332 _ _ _ w376 _ w418 _]
          tunnel: w234 -> [w259 w265 w271 w273 w275 w291 w301 w305 w316 w322 w337 w351 w359 w373 w385 w402 w423 w434]
          tunnel: [w238 w269 w271 w273 w280 w295 w300 w304 w308 w324 w339 w354 w356 w373 w381 w401 w419 w435] -> w236
          tunnel: w232 -> [w251 w268 w270 w272 w281 w296 w302 w303 w312 w319 w334 w352 w358 w372 w380 w399 w408 w432]
          tunnel: [w250 w266 w270 w272 w281 w296 w302 w303 w312 w317 w333 w352 w358 w372 w380 w399 w408 w432] -> w231
          tunnel: [_ _ _ _ _ _ _ _ _ _ _ _ _ _ _ _ w417 _] -> w230
          tunnel: w228 -> [_ _ _ _ _ _ _ _ w315 w323 w338 _ _ _ w379 _ w415 _]
          tunnel: w226 -> [w246 _ _ _ w282 w294 w298 _ _ _ _ _ _ _ w378 w397 w410 w431]
          tunnel: [_ _ _ _ _ _ _ _ _ _ _ _ _ _ _ _ w413 _] -> w225
          tunnel: w223 -> [_ _ _ _ _ _ _ _ w306 _ _ w346 w355 _ _ _ w407 _]
          frame "Initialize" {
            w243 = "Initial Message" ("Initial Message")
            # "#CodeNeeded - Initialize the appearance of the front panel."
            # "#CodeNeeded - Initialize your state data here."
            # "Initialize - Any operation that needs to be done before the module can receive messages. Synchronize Caller Events.vi will inform Start Module.vi that the module has launched and is ready to receive messages. Module Did Init.vi will broadcast that the module initialized."
            n107 = call "Synchronize Caller Events.vi"("error in"=w259, "Module Admin"=w246) -> ("error out"=w258:errorcluster, "Module Admin out"=w245:refnum<class "Delacor_lib_QMH_Cloneable Module Admin.lvclass">)  [unwired: 8 in]
            n108 = property on="Property Node" class="Mod Admin"(reference=w245) -> ("Accessors:Module ID"=w237:i32, "Accessors:External Launch"=w247:bool)  [unwired: 1 in, 2 out]
            n109 = call "Module Name--constant.vi"("Module ID"=w237) -> ("Module Name"=w255:string)  [unwired: 10 in]
            n110 = property on="Property Node" class="VI"("Front Panel.Title"=w255) -> (reference out=w257:refnum<vi>, error out=w261:errorcluster)  [unwired: 2 in]
            n111 = Select(t=T25."Hidden" ("State"), s=w247, f=T25."Standard" ("State")) -> (s? t:f=w252:T25)
            n112 = invoke on="Invoke Node" class="VI" method="FP.Open"(reference=w257, error in=w261, "State"=w252) -> (reference out=w256:refnum<vi>, error out=w260:errorcluster)  [unwired: 2 in, 3 out]
            n113 = call "Module Name--constant.vi"("Module ID"=w237) -> ("Module Name"=w248:string)  [unwired: 10 in]
            n114 = Bundle By Name(cluster=w251, "Status"=w243) -> (w250:T27)
            n115 = invoke on="Invoke Node" class="VI" method="FP.Center"(reference=w256, error in=w260) -> ()  [unwired: 1 in, 3 out]
            n116 = property on="Pane" class="Pane"("Origin"=T24 {"Horizontal"=0, "Vertical"=0}) -> ()  [unwired: 2 in, 2 out]
            n117 = call "Module Did Init.vi"("error in"=w258, "Initialized?"=TRUE, "Origin"=w248, "Module ID"=w237) -> ("error out"=w242:errorcluster)  [unwired: 7 in]
            n118 = call "Get Module Execution Status.vi"("Module ID"=w237) -> ()  [unwired: 10 in, 1 out]
            n119 = call-poly <vilib>:"Delacor_lib_QMH_Enqueue Message (poly).vi"("error in"=w242, "Message"="Init-1", "Message Queue in"=w241) -> ("error out"=w239:errorcluster)  [unwired: 7 in, 1 out]
            n120 = Merge Errors(w239) -> (w238:errorcluster)
            "Status" <- w243
          }
          frame "Init-1" {
            (unwired) "Send RT Initalizing Command" ("Message")
            # "Duplicate this frame when creating new messages.  Change this comment in the duplicated frame to describe this message."
            n121 = Bundle By Name(cluster=w268, "RT-IP"="Ip-Address") -> (w266:T27)
            n122 = call-poly <vilib>:"Delacor_lib_QMH_Enqueue Message (poly).vi"("error in"=w265, "Message"="Open TCP-Connection", "Message Queue in"=w263) -> ("error out"=w264:errorcluster)  [unwired: 7 in, 1 out]
            n123 = Merge Errors(w264) -> (w269:errorcluster)
          }
          frame "---Module Specific---" {
            # "Separator -- The following cases handle messages specific to this Module."
          }
          frame "-----Tx Data's to Other Module's-----" {
            # "Separator -- The following cases handle messages specific to this Module."
          }
          frame "Send Hardware Info" {
            n124 = Unbundle By Name(w281) -> ("RT-Data's.Hardware Information"=w274:variant, "Hardware Info Request Ref.Wait Notifier"=w279:refnum<notifier>, "Hardware Info Request Ref.wait for reply"=w278:bool)
            n125 = property class="Mod Admin"(reference=w282) -> ("Accessors:Module ID"=w285:i32)  [unwired: 1 in, 2 out]
            n126 = Bundle By Name(cluster=T26 {"Module ID"=-1, "Hardware Information"=variant(cluster{"Serial Hardware Info JSON Format":cluster{"Command":string, "SubCmd":string, "Channel":string[]}, "Hardware Info JSON Format":cluster{"Command":string, "SubCmd":string, "Input":string[], "Output":string[]}, "Hardware Info JSON Format":cluster{"Command":string, "SubCmd":string, "Input":string[], "Output":string[]}, "Ethernet IP Address JSON Format":cluster{"Command":string, "SubCmd":string, "IP":string[]}} {"Serial Hardware Info JSON Format"={"Command"="", "SubCmd"="", "Channel"=[]}, "Hardware Info JSON Format"={"Command"="", "SubCmd"="", "Input"=[], "Output"=[]}, "Hardware Info JSON Format"={"Command"="", "SubCmd"="", "Input"=[], "Output"=[]}, "Ethernet IP Address JSON Format"={"Command"="", "SubCmd"="", "IP"=[]}}), "error"={"status"=FALSE, "code"=0, "source"=""}} ("Hardware Info (Reply Payload)"), "Module ID"=w285, "Hardware Information"=w274, "error"=errorcluster {"status"=FALSE, "code"=0, "source"=""}) -> (w283:T26)
            n127 = case "DQMH_FIRE_NOTIFIER" shown="True" w278 {
              tunnel: w283 -> [_ w289]
              tunnel: w279 -> [_ w288]
              tunnel: [w286 w287] -> w276
              tunnel: w275 -> [w286 w287]
              frame False {
              }
              frame True {
                n128 = Send Notification(notification=w289, notifier=w288) -> ()  [unwired: 1 in, 2 out]
              }
            }
            n129 = call "Tx RT Hardware Info.vi"("Reply Payload"=w283) -> ()  [unwired: 10 in, 1 out]
            n130 = Merge Errors(w276) -> (w280:errorcluster)
          }
          frame "Send AI Info" {
            n131 = Unbundle By Name(w296) -> ("RT-Data's.AI-Data From RT--Cluster"=w293:T1)
            n132 = property on="Property Node" class="Mod Admin"(reference=w294) -> ("Accessors:Module ID"=w292:i32)  [unwired: 1 in, 2 out]
            n133 = call "AI-Info.vi"("error in"=w291, "AI-Info"=w293, "Module ID"=w292) -> ("error out"=w290:errorcluster)  [unwired: 8 in]
            n134 = Merge Errors(w290) -> (w295:errorcluster)
          }
          frame "Send DO Info" {
            n135 = Unbundle By Name(w302) -> ("RT-Data's.DO Info"=w299:T29)
            n136 = property on="Property Node" class="Mod Admin"(reference=w298) -> ("Accessors:Module ID"=w297:i32)  [unwired: 1 in, 2 out]
            n137 = call "DO Data's.vi"("DO Data's"=w299, "Module ID"=w297) -> ()  [unwired: 9 in, 1 out]
            n138 = Merge Errors(w301) -> (w300:errorcluster)
          }
          frame "---Copy This Frame---" {
            # "Duplicate this frame when creating new messages.  Change this comment in the duplicated frame to describe this message."
            n139 = Merge Errors(w305) -> (w304:errorcluster)
          }
          frame "Write Data To the RT" {
            # "This Request event will send the Data from the Host to Realtime Using TCP-IP Protocol."
            n140 = Variant To Data(error in=w316, type=T23 {"Module ID"=-1, "Data In"=""} ("Write Data To the RT Argument"), Variant=w315) -> (data=w313:T23, error out=w310:errorcluster)
            n141 = Unbundle By Name(w313) -> ("Data In"=w309:string)  [unwired: 1 out]
            n142 = call "TCP-Write.vi"("error in"=w310, "data in"=w309, "timeout ms (25000)"=500, "Module ID"=w306) -> ("error out"=w307:errorcluster)  [unwired: 7 in]
            n143 = Merge Errors(w307) -> (w308:errorcluster)
          }
          frame "Harware Info Request" {
            w320 = T31 {"Wait Notifier"=refnum, "wait for reply"=FALSE}  # Hardware Info
            n144 = Variant To Data(error in=w322, type=w320, Variant=w323) -> (data=w318:T31, error out=w321:errorcluster)
            n145 = Bundle By Name(cluster=w319, "Hardware Info Request Ref"=w318) -> (w317:T27)
            n146 = Merge Errors(w321) -> (w324:errorcluster)
          }
          frame "Decode TCP-Data" {
            w328 = T2 {"Interface"="CPU", "Command"="CPU Info", "SubCmd"="Monitor", "Data"=variant} ("TCP Tx-Rx Cluster")
            # "Duplicate this frame when creating new messages.  Change this comment in the duplicated frame to describe this message."
            n147 = Variant To Data(error in=w337, type="" ("TCP-IP Data Out"), Variant=w338) -> (data=w331:string, error out=w330:errorcluster)
            n148 = call <vilib>:"Unflatten From JSON String.vi"("Type and Defaults"=w328, "error in"=w330, "JSON String"=w331) -> ("error out"=w327:errorcluster, "Variant"=w329:variant)  [unwired: 7 in]
            n149 = Variant To Data(error in=w327, type=w328, Variant=w329) -> (data=w326:T2, error out=w325:errorcluster)
            "data" <- w326
            n150 = in-place {
              in-place-border: [w345] -> w335
              in-place-border: w325 -> [w344]
              in-place-border: w326 -> [w343]
              in-place-border: w332 -> [w340]
              n151 = in-place-cluster #1(w334) -> ("RT-Data's"=w342:T28)
              n152 = call "Decode TCP Data.vi"("TCP Rx-Tx Cluster In"=w343, "RT-Data's In"=w342, "Message Queue out"=w340, "error in"=w344) -> ("RT-Data's Out"=w341:T28, "error out"=w345:errorcluster)  [unwired: 10 in]
              n153 = in-place-cluster #1("RT-Data's"=w341) -> (w333:T27)
            }
            n154 = Merge Errors(w335) -> (w339:errorcluster)
          }
          frame "Open TCP-Connection" {
            # "Duplicate this frame when creating new messages.  Change this comment in the duplicated frame to describe this message."
            n155 = Unbundle By Name(w352) -> ("RT-IP"=w347:string)
            n156 = call "TCP-Open Connection.vi"("address"=w347, "remote port"=u16 6001, "error in"=w351, "timeout ms (60000)"=5000, "local port (0)"=u16 0, "Module ID"=w346) -> ("error out"=w350:errorcluster)  [unwired: 5 in]
            n157 = Merge Errors(w350) -> (w354:errorcluster)
          }
          frame "Send RT Initalizing Command" {
            # "Separator -- The following cases handle messages specific to this Module."
            n158 = for {
              N: 6 -> [_]
              tunnel: w355 -> [w365]
              shift-right: [w362] -> w357
              shift-left: w359 -> [w366]
              i -> [w361]
              n159 = call "Send Channel Configuration (SubVI).vi"("error in"=w366, "Operation Index"=w361) -> ("error out"=w364:errorcluster, "Command Data"=w363:string[])  [unwired: 8 in]
              n160 = for {
                tunnel: w365 -> [w371]
                tunnel: w363 -> [w368] mode=indexing
                shift-right: [w370] -> w362
                shift-left: w364 -> [w367]
                n161 = call "TCP-Write.vi"("error in"=w367, "data in"=w368, "timeout ms (25000)"=1000, "Module ID"=w371) -> ("error out"=w370:errorcluster)  [unwired: 7 in]
              }
            }
            n162 = Merge Errors(w357) -> (w356:errorcluster)
          }
          frame "---Exit and Error Handling---" {
            # "Separator - the following cases handle errors and exit messages."
          }
          frame "Error" {
            # "#CodeRecommended - If the module is running in standalone mode (External Launch = FALSE), this code will pop up an error dialog and call the 'Exit' message if an error occurs. Add more fine-grained error management here."
            # "Error - Check the error message data and respond accordingly. This message is sent by the \"Error Handler\" VIs at the end of each loop in this application."
            n163 = Variant To Data(error in=w385, type=errorcluster {"status"=FALSE, "code"=0, "source"=""} ("error constant"), Variant=w379) -> (data=w374:errorcluster, error out=w383:errorcluster)
            n164 = property on="Property Node" class="Mod Admin"(reference=w378) -> ("Accessors:External Launch"=w377:bool, "Accessors:Module ID"=w375:i32)  [unwired: 1 in, 2 out]
            n165 = local write "error out"(w374) -> ()
            n166 = call "Error Reported.vi"("Error"=w374, "Module ID"=w375) -> ()  [unwired: 9 in, 1 out]
            n167 = case shown="False" w377 {
              tunnel: [w390 _] -> w382
              tunnel: w376 -> [w388 _]
              tunnel: w374 -> [w389 _]
              frame False {
                n168 = disable-structure shown="Default" {
                  disable-tunnel: w389 -> [w391 _]
                  frame condition #0 (active) {
                    # "If the module is running standalone, then pop up an error dialog and call the \"Exit\" message."
                    n169 = call <vilib>:"Simple Error Handler.vi"("error in (no error)"=w391) -> ()  [unwired: 4 in, 5 out]
                  }
                  frame condition #1 {
                    # "To prevent the Simple Error Handler VI from being loaded (e.g. when deploying to a Real-Time target), add the Conditional Disable Symbol \"DQMH_Disable_SEH\" to your project and set it to TRUE."
                  }
                }
                n170 = call-poly <vilib>:"Delacor_lib_QMH_Enqueue Message (poly).vi"("Priority Message? (F)"=TRUE, "Message"="Exit", "Message Queue in"=w388) -> ("error out"=w390:errorcluster)  [unwired: 7 in, 1 out]
              }
              frame True {
                # "If the module was launched externally, calling the Error Reported broadcast VI is the only action performed by the \"Error\" message. The module's caller can then process the error appropriately."
              }
            }
            n171 = Merge Errors(w383, w382) -> (w381:errorcluster)
          }
          frame "Simulate MHL Error" {
            # "#DQMH_HowTo The 'Simulate MHL Error' button  illustrates how the MHL handles errors. This event is instructional in nature and can be removed."
            # "Simulate an error occurring at the MHL"
            n172 = property on="Property Node" class="Mod Admin"(reference=w397) -> ("Accessors:Module ID"=w398:i32)  [unwired: 1 in, 2 out]
            n173 = call "Module Name--constant.vi"("Module ID"=w398) -> ("Module Name"=w393:string)  [unwired: 10 in]
            n174 = Format Into String(format string="Simulated error originating at Message Handling Loop in %s", w393) -> (resulting string=w394:string)  [unwired: 2 in, 1 out]
            n175 = call <vilib>:"Error Cluster From Error Code.vi"("show call chain? (False)"=TRUE, "error message (\"\")"=w394, "error code (0)"=5001) -> ("error out"=w400:errorcluster)  [unwired: 6 in]
            n176 = Merge Errors(w402, w400) -> (w401:errorcluster)
          }
          frame "Exit" {
            w416 = 91  # 91: not all Exit messages will have an argument
            w417 = TRUE  # Stop the VI
            # "Release the message queue reference"
            # "Exit - Exit the application."
            n177 = Variant To Data(error in=w423, type=T22 {"Module ID"=-1, "Origin"="", "Exit via Stop Module Req?"=FALSE, "Wait for Module to stop?"=FALSE} ("Stop Argument"), Variant=w415) -> (data=w412:T22, error out=w420:errorcluster)
            n178 = call <vilib>:"Clear Errors.vi"("error in (no error)"=w420, "specific error code to clear (0: all)"=w416) -> ("error out"=w422:errorcluster)  [unwired: 4 in, 1 out]
            n179 = call <vilib>:"Clear Errors.vi"() -> ("error out"=w405:errorcluster)  [unwired: 6 in, 1 out]
            n180 = call "Stop Module.vi"("error in"=w405, "Module ID"=w407) -> ("error out"=w406:errorcluster)  [unwired: 9 in]
            n181 = property on="Property Node" class="Mod Admin"(reference=w410) -> ("Accessors:Module ID"=w409:i32)  [unwired: 1 in, 2 out]
            n182 = call <vilib>:"Clear Errors.vi"("error in (no error)"=w406) -> ("error out"=w403:errorcluster)  [unwired: 5 in, 1 out]
            n183 = call-dynamic "Delacor_lib_QMH_Release Message Queue.vi"("error in"=w422, "Message Queue"=w418) -> ("error out"=w421:errorcluster)  [unwired: 9 in]
            n184 = control-ref of="This VI"() -> (w411:refnum<vi>)
            n185 = call "Handle Exit.vi"("error in"=w403, "Stop Argument"=w412, "Module Admin in"=w410, "VI reference"=w411) -> ("error out"=w404:errorcluster, "Wait for Stop?"=w413:bool)  [unwired: 6 in]
            n186 = Merge Errors(w421, w404) -> (w419:errorcluster)
            n187 = call "Error Reported.vi"("Error"=w419, "Module ID"=w409) -> ()  [unwired: 9 in, 1 out]
          }
          frame Default {
            # "'Default' case only runs if there is a message that isn't defined in any of the other cases.  Output a programming error."
            n188 = property on="Property Node" class="Mod Admin"(reference=w431) -> ("Accessors:Module ID"=w430:i32)  [unwired: 1 in, 2 out]
            n189 = call "Module Name--constant.vi"("Module ID"=w430) -> ("Module Name"=w424:string)  [unwired: 10 in]
            n190 = Format Into String(format string="The invalid message string \"%s\" was received in the Message Handling Loop for module \"%s\".", w425, w424) -> (resulting string=w427:string)  [unwired: 2 in, 1 out]
            n191 = call <vilib>:"Error Cluster From Error Code.vi"("show call chain? (False)"=TRUE, "error message (\"\")"=w427, "error code (0)"=1) -> ("error out"=w433:errorcluster)  [unwired: 6 in]
            n192 = Merge Errors(w434, w433) -> (w435:errorcluster)
          }
        }
        n193 = call-dynamic "Delacor_lib_QMH_Error Handler - Message Handling Loop.vi"("error in"=w236, "Message Queue in"=w227) -> ("dup error in"=w233:errorcluster)  [unwired: 8 in, 1 out]
      }
      n194 = call <vilib>:"Stop Helper Loop.vi"("Helper Loop Periodic Timing in"=w27) -> ()  [unwired: 1 out]
      n195 = Unregister For Events(event registration refnum=w31) -> ()  [unwired: 1 in, 1 out]
    }
    frame Error {
      n196 = call "Synchronize Caller Events.vi"("Module Admin"=w439) -> ("Module Admin out"=w438:refnum<class "Delacor_lib_QMH_Cloneable Module Admin.lvclass">)  [unwired: 9 in, 1 out]
      n197 = property on="Property Node" class="Mod Admin"(reference=w438) -> ("Accessors:Module ID"=w437:i32)  [unwired: 1 in, 2 out]
      n198 = call-dynamic "Delacor_lib_QMH_Release Message Queue.vi"("error in"=w445, "Message Queue"=w436) -> ("error out"=w444:errorcluster)  [unwired: 9 in]
      n199 = call "Module Name--constant.vi"("Module ID"=w437) -> ("Module Name"=w442:string)  [unwired: 10 in]
      n200 = Format Into String(format string="An error occurred during initialization. %s is no longer running.", w442) -> (resulting string=w440:string)  [unwired: 2 in, 1 out]
      n201 = call "Error Reported.vi"("Additional Information"=w440, "Error"=w444, "Module ID"=w437) -> ()  [unwired: 8 in, 1 out]
    }
  }
  n202 = Merge Errors(w17, w16) -> (w18:errorcluster)
  n203 = call "Close Module.vi"("error in"=w18, "Wait for stop?"=w5, "Module Admin in"=w7) -> ("error out"=w15:errorcluster, "External Launch"=w4:bool, "Module Admin out"=w6:refnum<class "Delacor_lib_QMH_Cloneable Module Admin.lvclass">)  [unwired: 6 in]
  n204 = Unregister For Events(event registration refnum=w11, error in=w15) -> (error out=w14:errorcluster)
  "error out" <- w14
  n205 = case "External Launch?" shown="True" w4 {
    tunnel: w14 -> [_ w446]
    frame False {
    }
    frame True {
      n206 = case shown="No Error" w446 {
        frame No Error {
          n207 = invoke class="VI" method="FP.Close"() -> ()  [unwired: 3 in, 3 out]
        }
        frame Error {
          n208 = invoke class="VI" method="FP.Open"("Activate"=TRUE ("Activate?")) -> ()  [unwired: 4 in, 5 out]
        }
      }
    }
  }
  n209 = local write "Module Admin"(w6) -> ()
